vi "运维调试_氨氮.vi"() -> ()   [LabVIEW 2016, in "氨氮.lvlib"]
uses:
  <vilib>/Utility/miscctls.llb/LVPointTypeDef.ctl
  <vilib>/Utility/config.llb/NI_LVConfig.lvlib
panel:
  in  "质控参数设置":bool
  out "字符串":string
  in  "氨氮自动测试量程配置":T1
  out "ADC":sgl
  out "温度2":sgl
  out "温度1":sgl
  out "固件版本号":string
  in  "数组":string[](array[string])
  in  "备用系数写入":bool
  in  "备用系数读取":bool
  in  "备用系数":T2
  in  "量程切换阈值写入":bool
  in  "量程切换阈值读取":bool
  in  "量程切换阈值":cluster{"阈值":dbl, "标液浓度":dbl}
  in  "参数下拉列表":enum16{"氨氮", "总磷"}(ring)
  in  "量程下拉列表":enum16{"低量程", "高量程"}(ring)
  in  "测量模式下拉列表":enum16{"水样测量", "空白核查", "跨度核查", "标样核查", "加标回收"}(ring)
  in  "公式":cluster{"X^2":dbl, "X":dbl, "b":dbl}
  in  "写公式":bool
  in  "读公式":bool
  in  "精度":dbl=4.0
  in  "样品5 F0":dbl
  in  "样品5 F1":dbl
  in  "样品4 F1":dbl
  in  "样品4 F0":dbl
  in  "样品3 F0":dbl
  in  "样品3 F1":dbl
  in  "样品2 F0":dbl
  in  "样品2 F1":dbl
  in  "样品1 F1":dbl
  in  "样品1 F0":dbl
  in  "method":u16(ring) items=["最小二乘", "最小绝对残差", "Bisquare"]
  in  "模型":enum32{"线性", "多项式"}(ring)
  out "r^2":dbl format="%.7g"
  out "拟合公式":string
  in  "样品2启用":bool
  in  "样品5启用":bool
  in  "样品4启用":bool
  in  "样品3启用":bool
  in  "样品1启用":bool
  in  "标液浓度5":dbl
  in  "测量吸光度5":dbl
  in  "标液浓度4":dbl
  in  "测量吸光度4":dbl
  in  "标液浓度3":dbl
  in  "测量吸光度3":dbl
  in  "标液浓度2":dbl
  in  "测量吸光度2":dbl
  in  "测量吸光度1":dbl
  in  "标液浓度1":dbl
  out "XY图":cluster{"X Values":dbl[], "Y Values":dbl[]}[](graph)
  in  "返回":bool
  in  "设置":bool
  out "序列号":string="序列号"
  out "氨氮测量数据":T3(xcontrol)
  out "集成报警信息":string
  out "定时启动":bool
  out "总磷总氮运行状态":T4(xcontrol)
  in  "停止":bool
  in  "手动启动":bool
  in  "单步测试":bool
  in  "总磷氨氮调试":u16[](xcontrol)
  out "F3":sgl format="%#.6f"
  out "F2":sgl format="%#.6f"
  out "F1":sgl format="%#.6f"
  out "F0":sgl format="%#.6f"
  out "多列列表框":i32(listbox)
  # "参数设置"
  # "标液浓度"
  # "F0"
  # "F1"
  # "吸光值显示"
  # "样品一"
  # "辅\n助\n计\n算\n区"
  # "样品二"
  # "样品三"
  # "样品四"
  # "样品五"
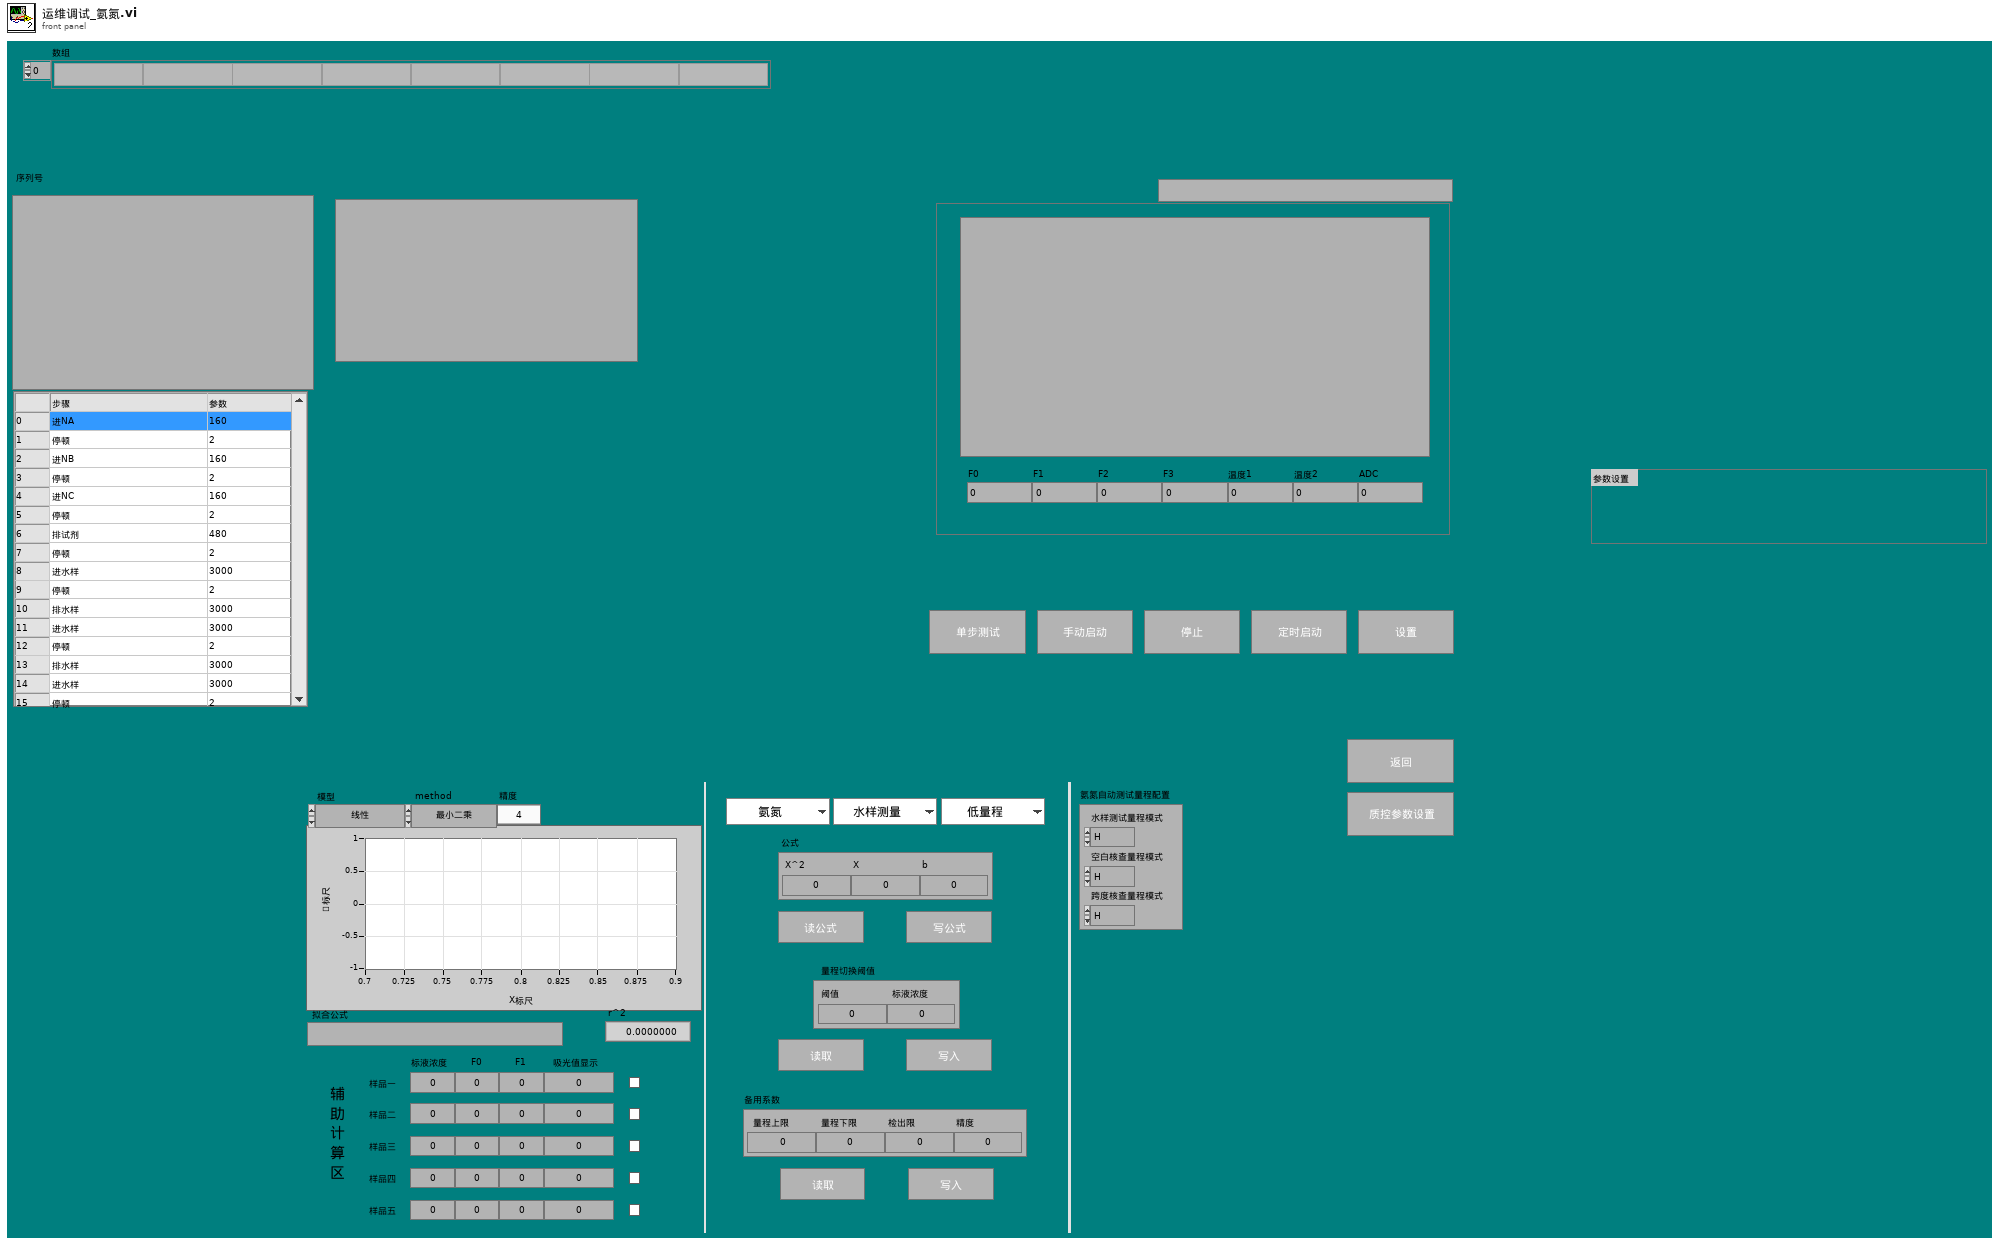
[diagram p1: front panel]
types:
  T1 = cluster{"水样测试量程模式":enum16{"H", "L", "AUTO"}, "空白核查量程模式":enum16{"H", "L", "AUTO"}, "跨度核查量程模式":enum16{"H", "L", "AUTO"}}
  T2 = cluster{"量程上限":dbl, "量程下限":dbl, "检出限":dbl, "精度":dbl}
  T3 = cluster{"flowid":u16, "测量精度":u16, "测量数据区":cluster{"因子编码":u32, "单位":u16, "标样参考值":sgl, "水样数据时间":timestamp, "水样实测值":sgl, "水样数据标识":string, "标样数据时间":timestamp, "标样实测值":sgl, "标样数据标识":string, "空白数据时间":timestamp, "空白实测值":sgl, "空白数据标识":string, "零点核查数据时间":timestamp, "零点核查实测值":sgl, "零点核查数据标识":string, "跨度核查数据时间":timestamp, "跨度核查实测值":sgl, "跨度核查数据标识":string, "加标回收数据时间":timestamp, "加标回收实测值":sgl, "加标回收数据标识":string, "平行样数据时间":timestamp, "平行样实测值":sgl, "平行样数据标识":string}}
  T4 = cluster{"系统时间":timestamp, "工作状态":enum16{"空闲", "水样测试", "标样核查", "零点核查", "跨度核查", "空白测试", "平行样测试", "加标回收", "空白校准", "标样校准", "初始化（清洗）"}, "测量模式":enum16{"待机", "连续模式", "周期模式", "定点模式", "受控模式", "手动模式"}, "告警代码":enum16{"无告警", "缺试剂告警", "缺水样告警", "缺蒸馏水告警", "缺标液告警", "仪表漏液告警", "标定异常告警", "超量程告警", "加热异常", "低试剂预警", "超上限告警", "超下限告警", "仪表内部其他异常", "滴定异常告警", "电极异常告警", "量程切换告警", "参数设置告警", "PH电极电位异常", "电导率电极异常", "浊度光度异常", "溶解氧电极异常", "溶解氧光强异常", "温度异常告警", "PH异常告警", "溶解氧异常告警", "电导率异常告警", "浊度异常告警", "叶绿素异常告警", "藻密度异常告警", "蓝绿藻异常告警", "ORP异常告警", "氨氮异常告警", "清洁刷异常告警", "SD卡异常告警", "蓝牙异常告警", "Wifi异常告警", "流程异常告警"}, "故障代码":enum16{"无故障", "电机故障", "温度故障", "通讯故障", "滴定故障"}, "日志代码":u16, "软件版本":u16, "F0":sgl, "F1":sgl, "F2":sgl, "F3":sgl, "T":sgl, "H":sgl, "id":u16, "flowid":u16, "量程":u16, "总磷控温温度1":sgl, "营养盐控温温度2":sgl, "ADC":sgl}
  T5 = cluster{"站号":u16, "量程切换":enum32{"H", "L", "AUTO"}, "控制命令":enum16{"启动测量", "标样核查", "零点核查", "跨度核查", "空白测试", "平行样测试", "加标回收", "空白校准", "标样校准", "初始化（清洗）", "停止测试", "仪器重启", "校时", "模式设置", "测量间隔设置"}, "模式设置":enum16{"待机", "连续模式", "周期模式", "定点模式", "受控模式", "手动模式"}, "测量间隔":u16}
  T6 = enum16{"启动测量", "标样核查", "零点核查", "跨度核查", "空白测试", "平行样测试", "加标回收", "空白校准", "标样校准", "初始化（清洗）", "停止测试", "仪器重启", "校时", "模式设置", "测量间隔设置"}
  T7 = cluster{"仪器测试类型":enum16{"水样测试", "标样核查", "空白测试", "跨度核查"}, "周期设置类型":enum16{"定点启动", "间隔启动"}, "定时功能启用":bool, "定时间隔":dbl, "24H周期设置":bool[]}
  T8 = enum32{"Bad", "Idle", "Run top level", "Running"}
  T9 = typedef "LVDateTimeRec.ctl" = cluster{"秒数的小数部分":dbl, "秒":i32, "分":i32, "时":i32, "日":i32, "月":i32, "年":i32, "天数（周）":i32, "天数（年）":i32, "DST":i32}
  T10 = typedef "LVPointTypeDef.ctl" = cluster{"Horizontal":i16, "Vertical":i16}
  T11 = cluster{"因子编码":u32, "单位":u16, "标样参考值":sgl, "水样数据时间":timestamp, "水样实测值":sgl, "水样数据标识":string, "标样数据时间":timestamp, "标样实测值":sgl, "标样数据标识":string, "空白数据时间":timestamp, "空白实测值":sgl, "空白数据标识":string, "零点核查数据时间":timestamp, "零点核查实测值":sgl, "零点核查数据标识":string, "跨度核查数据时间":timestamp, "跨度核查实测值":sgl, "跨度核查数据标识":string, "加标回收数据时间":timestamp, "加标回收实测值":sgl, "加标回收数据标识":string, "平行样数据时间":timestamp, "平行样实测值":sgl, "平行样数据标识":string}
  T12 = enum16{"空闲", "水样测试", "标样核查", "零点核查", "跨度核查", "空白测试", "平行样测试", "加标回收", "空白校准", "标样校准", "初始化（清洗）"}
  T13 = cluster{"启动模式":enum16{"标液测量", "水样测量", "零液测量", "盲样测量", "加标回收"}, "启动参数":u16, "量程":enum16{"低量程", "高量程"}}
  T14 = cluster{"时间标识":timestamp, "设备":string, "日志信息":string, "流程参数":string}
  T15 = cluster{"时间标识":timestamp, "设备":string, "日志信息":string}
  T16 = enum16{"无告警", "缺试剂告警", "缺水样告警", "缺蒸馏水告警", "缺标液告警", "仪表漏液告警", "标定异常告警", "超量程告警", "加热异常", "低试剂预警", "超上限告警", "超下限告警", "仪表内部其他异常", "滴定异常告警", "电极异常告警", "量程切换告警", "参数设置告警", "PH电极电位异常", "电导率电极异常", "浊度光度异常", "溶解氧电极异常", "溶解氧光强异常", "温度异常告警", "PH异常告警", "溶解氧异常告警", "电导率异常告警", "浊度异常告警", "叶绿素异常告警", "藻密度异常告警", "蓝绿藻异常告警", "ORP异常告警", "氨氮异常告警", "清洁刷异常告警", "SD卡异常告警", "蓝牙异常告警", "Wifi异常告警", "流程异常告警"}
  T17 = typedef "LVRowAndColumnUnsignedTypeDef.ctl" = cluster{"Row":u32, "Column":u32}
  T18 = typedef "NI_LVConfig.lvlib/Config Data RefNum.ctl" = refnum<k1>
  T19 = cluster{"XY图":cluster{"X Values":dbl[], "Y Values":dbl[]}[], "标液浓度1":dbl, "测量吸光度1":dbl, "测量吸光度2":dbl, "标液浓度2":dbl, "测量吸光度3":dbl, "标液浓度3":dbl, "测量吸光度4":dbl, "标液浓度4":dbl, "测量吸光度5":dbl, "标液浓度5":dbl, "样品1启用":bool, "样品3启用":bool, "样品4启用":bool, "样品5启用":bool, "样品2启用":bool, "拟合公式":string, "r^2":dbl, "模型":enum32{"线性", "多项式"}, "method":u16, "样品1 F0":dbl, "样品1 F1":dbl, "样品2 F1":dbl, "样品2 F0":dbl, "样品3 F1":dbl, "样品3 F0":dbl, "样品4 F0":dbl, "样品4 F1":dbl, "样品5 F1":dbl, "样品5 F0":dbl, "精度":dbl}
  T20 = cluster{"跨度值":dbl, "零点标准液浓度":dbl, "跨度标准液浓度":dbl, "标准液标准浓度":dbl}
  T21 = cluster{"确定":bool, "跨度值":dbl, "零点标准液浓度":dbl, "跨度标准液浓度":dbl, "标准液标准浓度":dbl}
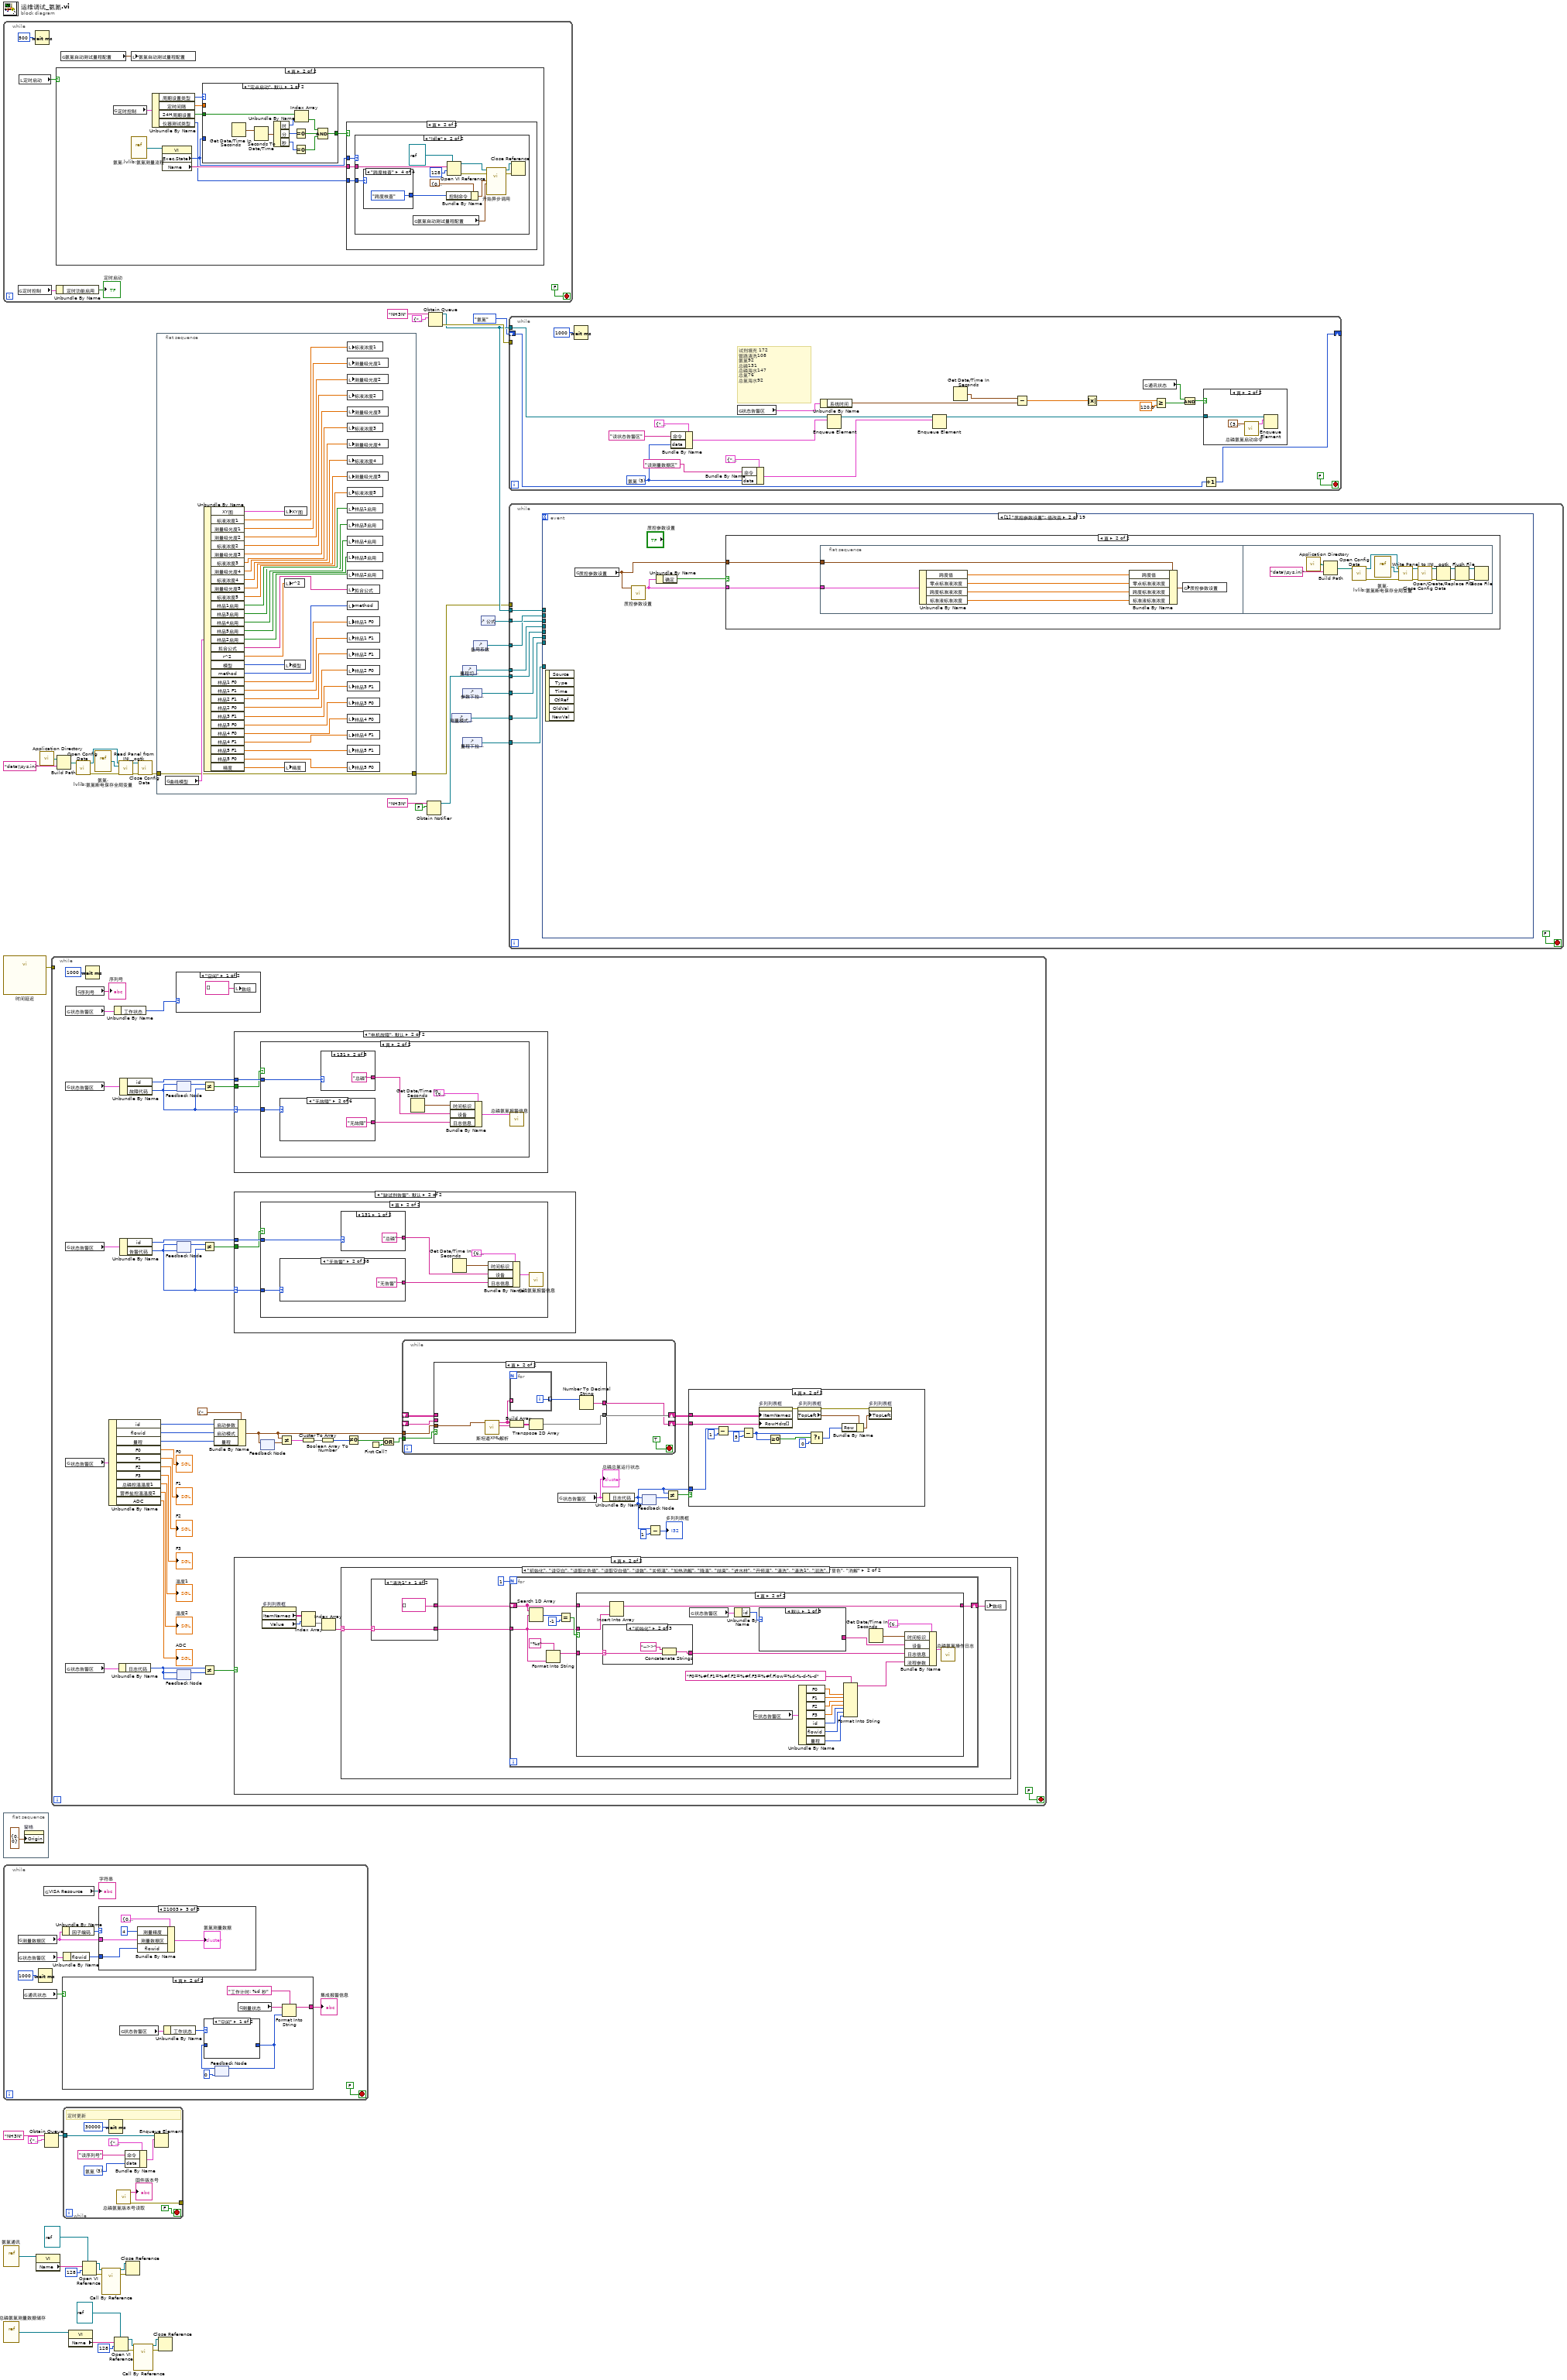
[diagram p0: block diagram]
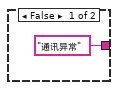
[diagram p2: hidden frame]
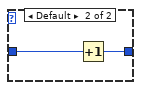
[diagram p3: hidden frame]
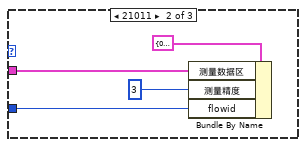
[diagram p5: hidden frame]
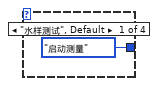
[diagram p9: hidden frame]
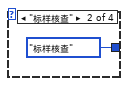
[diagram p10: hidden frame]
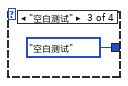
[diagram p11: hidden frame]
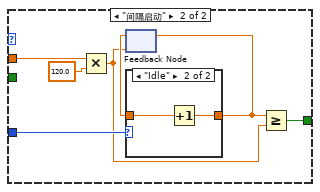
[diagram p12: hidden frame]
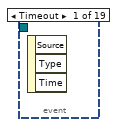
[diagram p14: hidden frame]
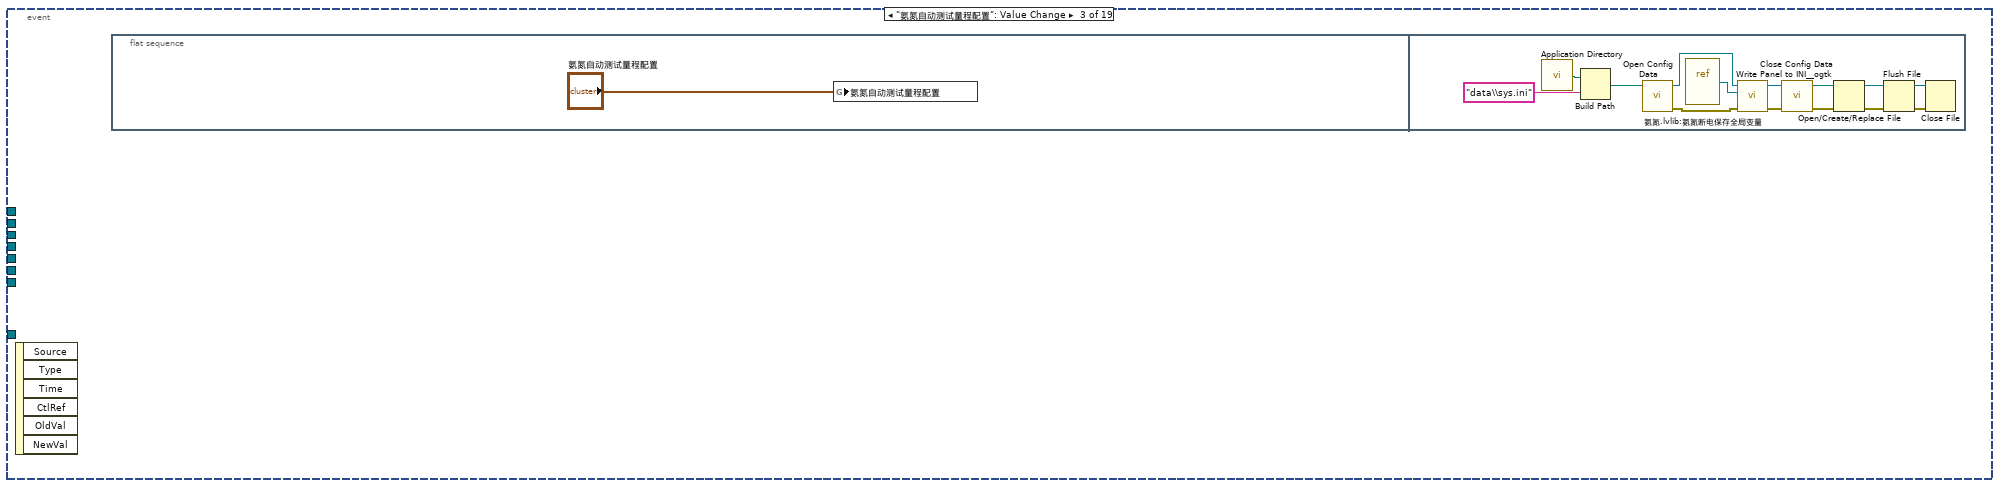
[diagram p16: hidden frame]
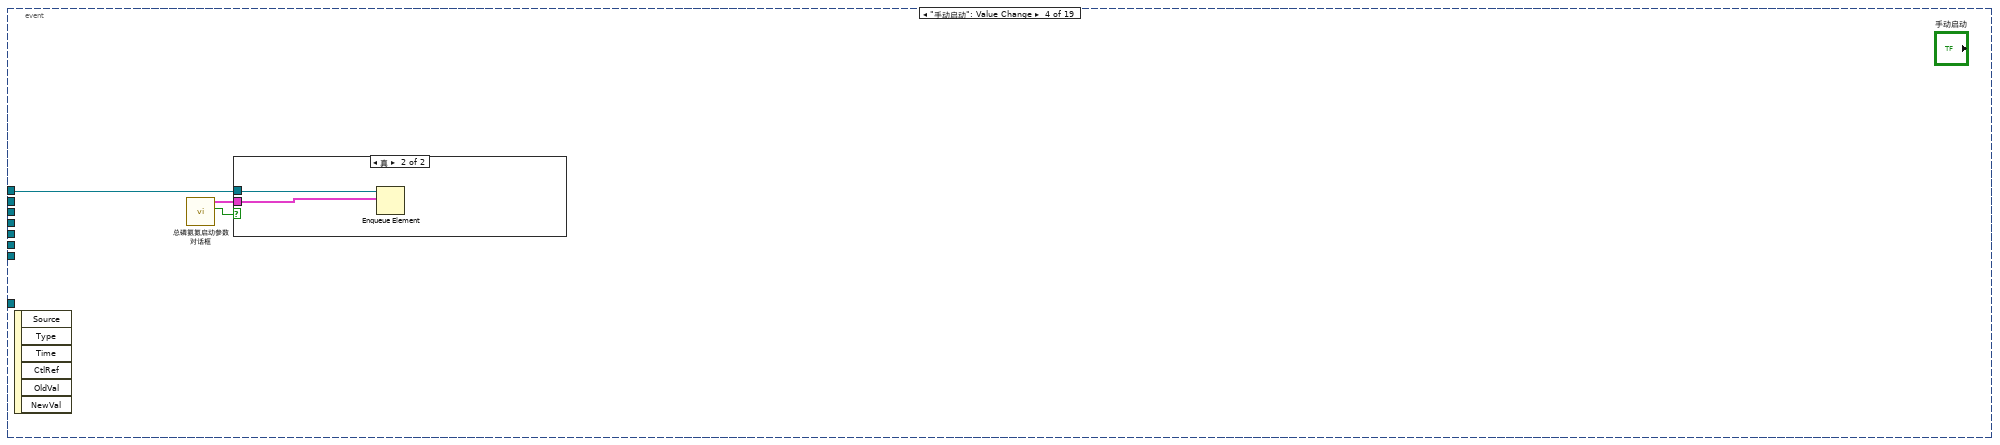
[diagram p17: hidden frame]
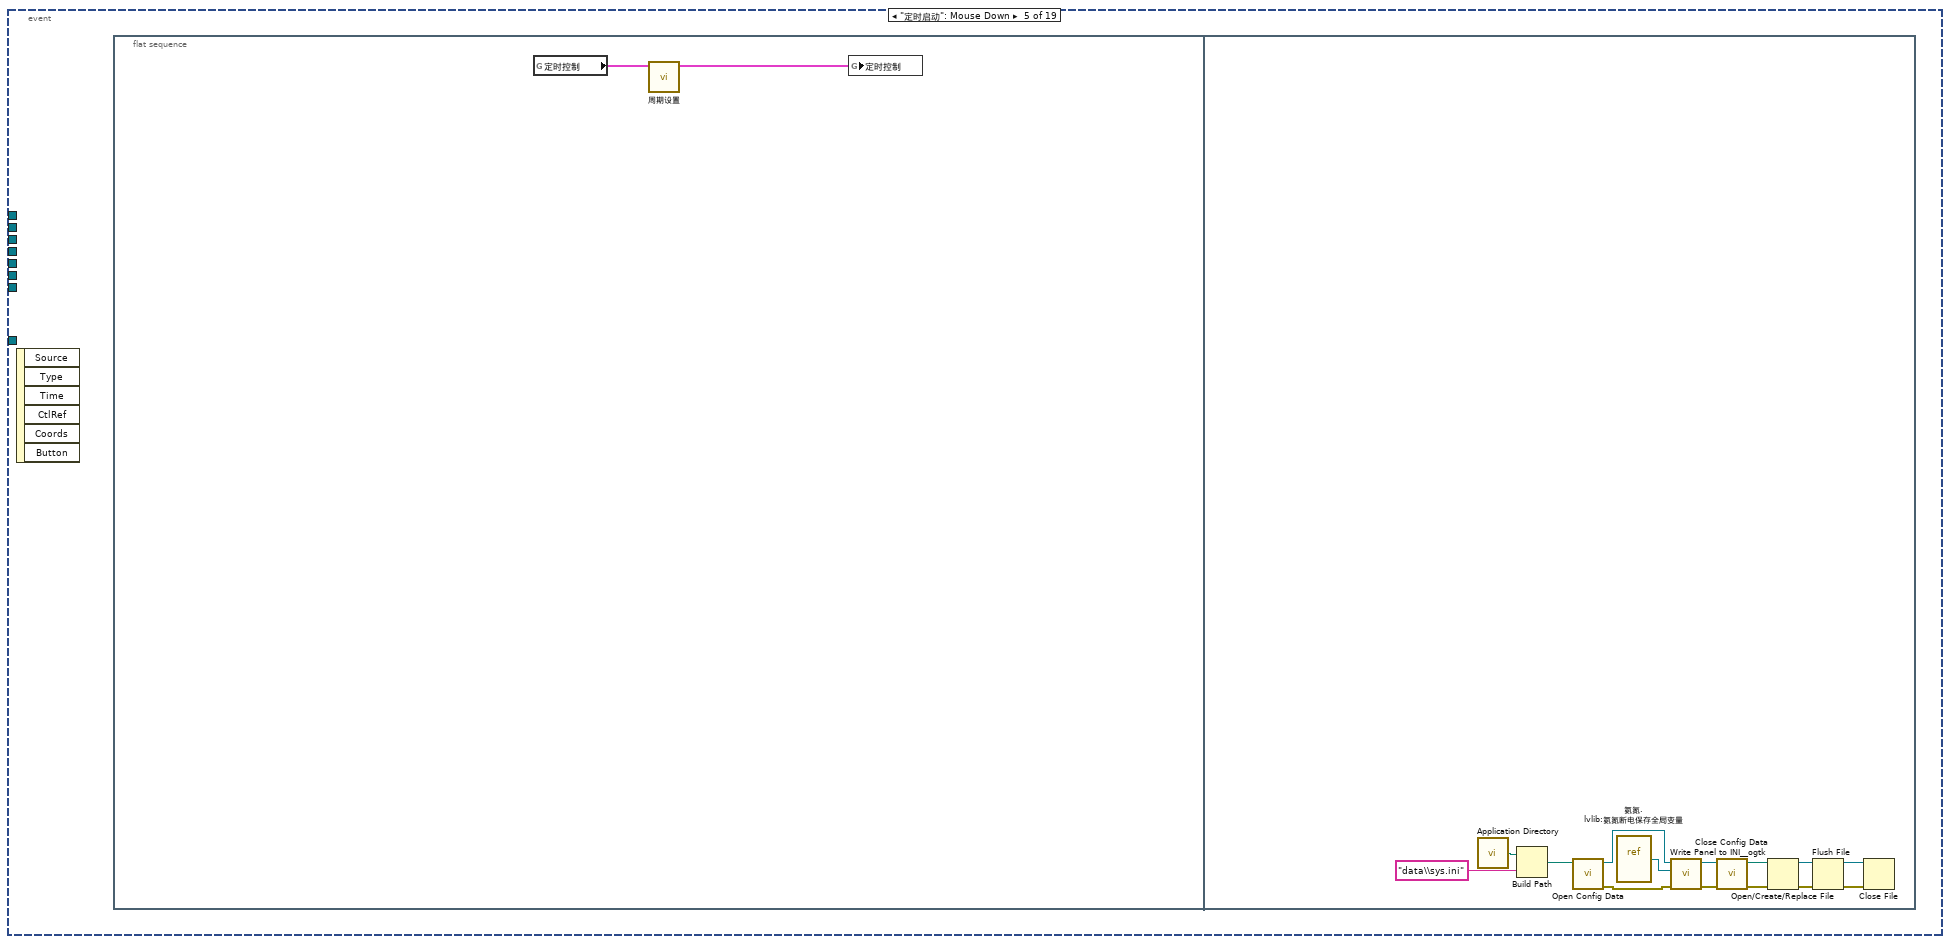
[diagram p19: hidden frame]
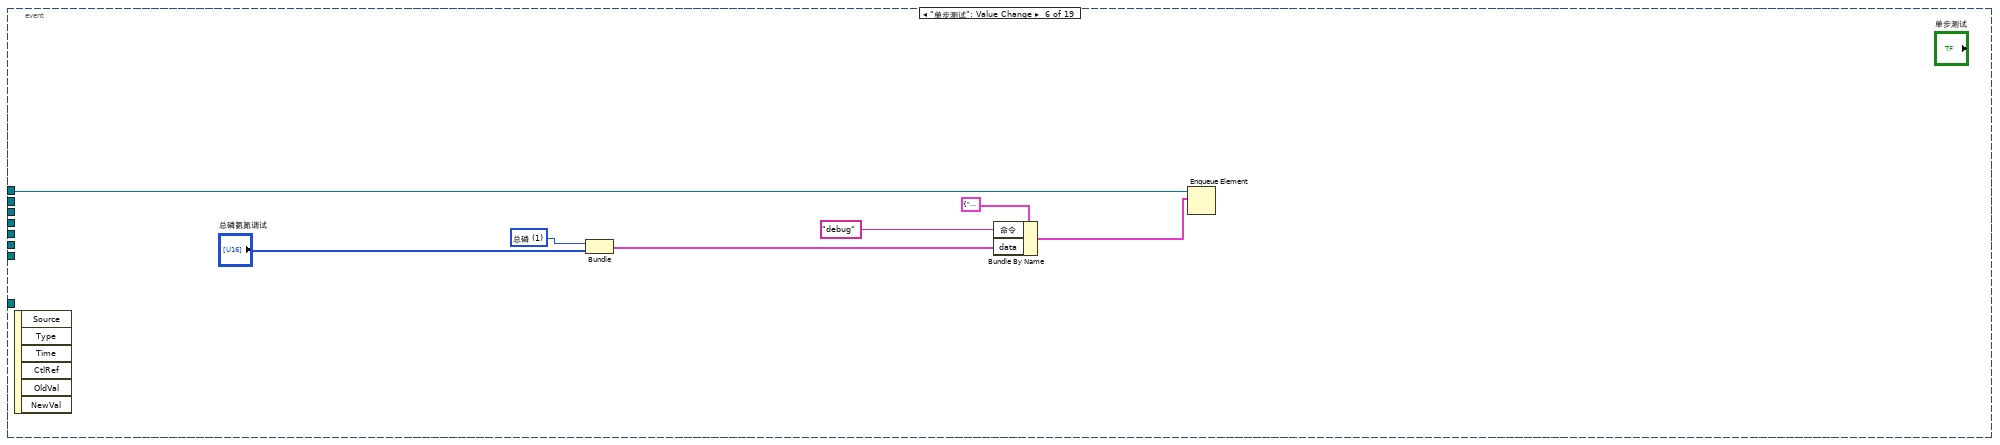
[diagram p20: hidden frame]
diagram:
  n1 = while {
    stop <- FALSE stop-if-true
    n2 = global read "氨氮断电保存全局变量.vi" "定时控制"() -> (w47:T7)
    n3 = local read "定时启动"() -> (w48:bool)
    n4 = Wait (ms)(milliseconds to wait=u32 500 ("等待时间（毫秒）")) -> ()  [unwired: 1 out]
    n5 = case shown="真" w48 {
      frame False {
      }
      frame True {
        n6 = global read "氨氮断电保存全局变量.vi" "定时控制"() -> (w59:T7)
        n7 = vi-ref "氨氮.lvlib:氨氮测量流程.vi"() -> (w55:refnum<vi>)
        n8 = Unbundle By Name(w59) -> ("周期设置类型"=w58:enum16{"定点启动", "间隔启动"}, "定时间隔"=w57:dbl, "24H周期设置"=w56:bool[], "仪器测试类型"=w52:enum16{"水样测试", "标样核查", "空白测试", "跨度核查"})
        n9 = property class="VI"(reference=w55) -> ("Exec.State"=w51:T8, "Name"=w54:string)  [unwired: 1 in, 2 out]
        n10 = case shown="\"定点启动\", 默认" w58 {
          tunnel: w57 -> [_ w92]
          tunnel: w56 -> [w88 _]
          tunnel: w51 -> [_ w95]
          tunnel: [w87 w90] -> w53
          frame "定点启动", Default {
            n11 = Get Date/Time In Seconds() -> (seconds since 1Jan1904=w86:timestamp)
            n12 = Seconds To Date/Time(time stamp (now)=w86) -> (date time rec=w85:T9)  [unwired: 1 in]
            n13 = Unbundle By Name(w85) -> ("时"=w84:i32, "分"=w82:i32, "秒"=w83:i32)
            n14 = Equal To 0?(x=w82) -> (x = 0?=w80:bool)
            n15 = Equal To 0?(x=w83) -> (x = 0?=w79:bool)
            n16 = Index Array(array=w88, index=w84) -> (element=w81:bool)
            n17 = Compound Arithmetic op=AND ("复合运算")(w81, w80, w79) -> (w87:bool)
          }
          frame "间隔启动" {
            n18 = Multiply(x=w92, y=120.0) -> (x*y=w89:dbl)
            n19 = feedback #1(w89) -> (w94:dbl)
            n20 = case shown="\"Idle\"" w95 {
              tunnel: w94 -> [_ w97]
              tunnel: [_ w96] -> w93
              frame "Bad", Default {
              }
              frame "Idle" {
                n21 = Increment(x=w97) -> (x+1=w96:dbl)
              }
            }
            n22 = feedback-in #1(w93) -> ()
            n23 = Greater Or Equal?(x=w93, y=w89) -> (x >= y?=w90:bool)
          }
        }
        n24 = case shown="真" w53 {
          tunnel: w54 -> [_ w62]
          tunnel: w52 -> [_ w61]
          tunnel: w51 -> [_ w60]
          frame False {
          }
          frame True {
            n25 = case shown="\"Idle\"" w60 {
              tunnel: w62 -> [_ w69]
              tunnel: w61 -> [_ w65]
              frame "Bad", Default {
              }
              frame "Idle" {
                n26 = case shown="\"跨度核查\"" w65 {
                  tunnel: [T6."启动测量" ("控制命令") T6."标样核查" ("控制命令") T6."空白测试" ("控制命令") T6."跨度核查" ("控制命令")] -> w64
                  frame "水样测试", Default {
                  }
                  frame "标样核查" {
                  }
                  frame "空白测试" {
                  }
                  frame "跨度核查" {
                  }
                }
                n27 = global read "氨氮断电保存全局变量.vi" "氨氮自动测试量程配置"() -> (w63:T1)
                n28 = Bundle By Name(cluster=T5 {"站号"=0, "量程切换"=enum."H", "控制命令"=enum."启动测量", "模式设置"=enum."待机", "测量间隔"=0} ("参数"), "控制命令"=w64) -> (w66:T5)
                n29 = Open VI Reference(type specifier VI Refnum (for type only)=refnum<vi> refnum, vi path=w69, options=128 ("选项")) -> (vi reference=w70:refnum<vi>, error out=w71:errorcluster)  [unwired: 3 in]
                n30 = call-by-ref "开始异步调用"(reference=w70, error in=w71, "量程模式"=w63, "参数"=w66) -> (reference out=w72:refnum<vi>, error out=w73:errorcluster)  [unwired: 10 in]
                n31 = Close Reference(reference=w72, error in (no error)=w73) -> ()  [unwired: 1 out]
              }
            }
          }
        }
      }
    }
    n32 = Unbundle By Name(w47) -> ("定时功能启用"=→"定时启动":bool)
    n33 = global read "氨氮断电保存全局变量.vi" "氨氮自动测试量程配置"() -> (w45:T1)
    n34 = local write "氨氮自动测试量程配置"(w45) -> ()
  }
  n35 = call "时间延迟"() -> ("error out"=w17:errorcluster)  [unwired: 11 in]
  n36 = flat-sequence {
    frame #0 {
      n37 = property on="窗格" class="Pane"("Origin"=T10 {"Horizontal"=0, "Vertical"=0} ("原点")) -> ()  [unwired: 2 in, 2 out]
    }
  }
  n38 = while {
    stop <- FALSE stop-if-true
    n39 = global read "VAR总磷氨氮全局变量.vi" "测量数据区"() -> (w105:T11)
    n40 = global read "VAR总磷氨氮全局变量.vi" "状态告警区"() -> (w101:T4)
    n41 = global read "VAR总磷氨氮全局变量.vi" "通讯状态"() -> (w103:bool)
    n42 = Wait (ms)(milliseconds to wait=u32 1000 ("等待时间（毫秒）")) -> ()  [unwired: 1 out]
    n43 = global read "VAR总磷氨氮全局变量.vi" "VISA Resource"() -> (→"字符串":refnum<visa-resource-name>)
    n44 = Unbundle By Name(w105) -> ("因子编码"=w104:u32)
    n45 = case shown="真" w103 {
      tunnel: ["通讯异常" ("集成报警信息") w110] -> w102
      frame False {
      }
      frame True {
        n46 = global read "VAR总磷氨氮全局变量.vi" "状态告警区"() -> (w116:T4)
        n47 = Unbundle By Name(w116) -> ("工作状态"=w115:T12)
        n48 = feedback #2(0) -> (w113:i32)
        n49 = case shown="\"空闲\"" w115 {
          tunnel: w113 -> [_ w118]
          tunnel: [_ w117] -> w111
          frame "空闲" {
          }
          frame Default {
            n50 = Increment(x=w118) -> (x+1=w117:i32)
          }
        }
        n51 = feedback-in #2(w111) -> ()
        n52 = global read "VAR总磷氨氮全局变量.vi" "测量状态"() -> (w109:string)
        n53 = Format Into String(format string="工作计时: %d 秒" ("格式字符串"), initial string=w109, w111) -> (resulting string=w110:string)  [unwired: 1 in, 1 out]
      }
    }
    "集成报警信息" <- w102
    n54 = Unbundle By Name(w101) -> ("flowid"=w100:u16)
    n55 = case shown="21003" w104 {
      tunnel: w105 -> [_ w122 w127]
      tunnel: w100 -> [_ w120 w125]
      frame Default {
      }
      frame 21011 {
        n56 = Bundle By Name(cluster=T3 {"flowid"=0, "测量精度"=0, "测量数据区"={"因子编码"=0, "单位"=0, "标样参考值"=0.0, "水样数据时间"=timestamp(0 s since 1904-01-01), "水样实测值"=0.0, "水样数据标识"="", "标样数据时间"=timestamp(0 s since 1904-01-01), "标样实测值"=0.0, "标样数据标识"="", "空白数据时间"=timestamp(0 s since 1904-01-01), "空白实测值"=0.0, "空白数据标识"="", "零点核查数据时间"=timestamp(0 s since 1904-01-01), "零点核查实测值"=0.0, "零点核查数据标识"="", "跨度核查数据时间"=timestamp(0 s since 1904-01-01), "跨度核查实测值"=0.0, "跨度核查数据标识"="", "加标回收数据时间"=timestamp(0 s since 1904-01-01), "加标回收实测值"=0.0, "加标回收数据标识"="", "平行样数据时间"=timestamp(0 s since 1904-01-01), "平行样实测值"=0.0, "平行样数据标识"=""}} ("氨氮测量数据"), "测量数据区"=w122, "测量精度"=u16 3, "flowid"=w120) -> ()  [unwired: 1 out]
      }
      frame 21003 {
        n57 = Bundle By Name(cluster=T3 {"flowid"=0, "测量精度"=0, "测量数据区"={"因子编码"=0, "单位"=0, "标样参考值"=0.0, "水样数据时间"=timestamp(0 s since 1904-01-01), "水样实测值"=0.0, "水样数据标识"="", "标样数据时间"=timestamp(0 s since 1904-01-01), "标样实测值"=0.0, "标样数据标识"="", "空白数据时间"=timestamp(0 s since 1904-01-01), "空白实测值"=0.0, "空白数据标识"="", "零点核查数据时间"=timestamp(0 s since 1904-01-01), "零点核查实测值"=0.0, "零点核查数据标识"="", "跨度核查数据时间"=timestamp(0 s since 1904-01-01), "跨度核查实测值"=0.0, "跨度核查数据标识"="", "加标回收数据时间"=timestamp(0 s since 1904-01-01), "加标回收实测值"=0.0, "加标回收数据标识"="", "平行样数据时间"=timestamp(0 s since 1904-01-01), "平行样实测值"=0.0, "平行样数据标识"=""}} ("氨氮测量数据"), "测量精度"=u16 4, "测量数据区"=w127, "flowid"=w125) -> (→"氨氮测量数据":T3)
      }
    }
  }
  n58 = vi-ref "氨氮通讯.vi"() -> (w40:refnum<vi>)
  n59 = vi-ref "总磷氨氮测量数据储存.vi"() -> (w32:refnum<vi>)
  n60 = property class="VI"(reference=w40) -> ("Name"=w39:string)  [unwired: 1 in, 2 out]
  n61 = call <vilib>:"Application Directory.vi"() -> ("Application Directory"=w3:path)
  n62 = Obtain Queue(name (unnamed)="NH3N" ("名称（未命名）"), element data type=cluster{"命令":string, "data":variant} {"命令"="", "data"=variant}) -> (queue out=w14:refnum<queue>)  [unwired: 3 in, 2 out]
  n63 = while {
    tunnel: w17 -> [_]
    stop <- FALSE stop-if-true
    n64 = global read "VAR总磷氨氮全局变量.vi" "状态告警区"() -> (w139:T4)
    n65 = global read "VAR总磷氨氮全局变量.vi" "状态告警区"() -> (w144:T4)
    n66 = global read "VAR总磷氨氮全局变量.vi" "状态告警区"() -> (w149:T4)
    n67 = global read "VAR总磷氨氮全局变量.vi" "状态告警区"() -> (w161:T4)
    n68 = global read "VAR总磷氨氮全局变量.vi" "状态告警区"() -> (w136:T4)
    n69 = global read "VAR总磷氨氮全局变量.vi" "序列号"() -> (→"序列号":string)
    n70 = Wait (ms)(milliseconds to wait=u32 1000 ("等待时间（毫秒）")) -> ()  [unwired: 1 out]
    n71 = Unbundle By Name(w161) -> ("id"=w158:u16, "flowid"=w160:u16, "量程"=w159:u16, "F0"=→"F0":sgl, "F1"=→"F1":sgl, "F2"=→"F2":sgl, "F3"=→"F3":sgl, "总磷控温温度1"=→"温度1":sgl, "营养盐控温温度2"=→"温度2":sgl, "ADC"=→"ADC":sgl)
    n72 = Unbundle By Name(w139) -> ("工作状态"=w138:T12)
    n73 = Unbundle By Name(w136) -> ("日志代码"=w135:u16)
    n74 = Unbundle By Name(w144) -> ("id"=w143:u16, "故障代码"=w140:enum16{"无故障", "电机故障", "温度故障", "通讯故障", "滴定故障"})
    n75 = Unbundle By Name(w149) -> ("id"=w148:u16, "告警代码"=w145:T16)
    n76 = case shown="\"空闲\"" w138 {
      frame "空闲" {
        n77 = local write "数组"(string[] [] ("数组")) -> ()
      }
      frame "水样测试", Default {
      }
    }
    n78 = feedback #3(w140) -> (w141:enum16{"无故障", "电机故障", "温度故障", "通讯故障", "滴定故障"})
    n79 = feedback-in #3(w140) -> ()
    n80 = feedback #4(w145) -> (w146:T16)
    n81 = feedback-in #4(w145) -> ()
    n82 = feedback #5(w135) -> (w137:u16)
    n83 = feedback-in #5(w135) -> ()
    n84 = Not Equal?(x=w141, y=w140) -> (x != y?=w142:bool)
    n85 = Not Equal?(x=w146, y=w145) -> (x != y?=w147:bool)
    n86 = Not Equal?(x=w135, y=w137) -> (x != y?=w134:bool)
    n87 = Bundle By Name(cluster=T13 {"启动模式"=enum."加标回收", "启动参数"=1, "量程"=enum."低量程"} ("参数簇"), "启动参数"=w158, "启动模式"=w160, "量程"=w159) -> (w151:T13)
    n88 = case shown="\"电机故障\", 默认" w140 {
      selector: w140 -> [_ w229]
      tunnel: w143 -> [_ w230]
      tunnel: w142 -> [_ w228]
      frame "无故障" {
      }
      frame "电机故障", Default {
        n89 = case shown="真" w228 {
          tunnel: w230 -> [_ w237]
          tunnel: w229 -> [_ w232]
          frame False {
          }
          frame True {
            n90 = case shown="\"无故障\"" w232 {
              selector: w232 -> [w239 _ _ _ _ _]
              tunnel: [w238 "无故障" "电机故障" "温度故障" "通讯故障" "滴定故障"] -> w231
              frame Default {
                n91 = Format Into String(format string="%d" ("格式字符串"), initial string="未知" ("工作状态"), w239) -> (resulting string=w238:string)  [unwired: 1 in, 1 out]
              }
              frame "无故障" {
              }
              frame "电机故障" {
              }
              frame "温度故障" {
              }
              frame "通讯故障" {
              }
              frame "滴定故障" {
              }
            }
            n92 = case shown="131" w237 {
              tunnel: [_ "总磷" ("table输入") "氨氮" ("table输入")] -> w233
              frame Default {
              }
              frame 131 {
              }
              frame 92 {
              }
            }
            n93 = Get Date/Time In Seconds() -> (seconds since 1Jan1904=w234:timestamp)
            n94 = Bundle By Name(cluster=T15 {"时间标识"=timestamp(0 s since 1904-01-01), "设备"="", "日志信息"=""} ("data in"), "时间标识"=w234, "设备"=w233, "日志信息"=w231) -> (w235:T15)
            n95 = call "总磷氨氮报警信息.vi"("data in"=w235) -> ()  [unwired: 11 in]
          }
        }
      }
    }
    n96 = case shown="\"缺试剂告警\", 默认" w145 {
      selector: w145 -> [_ w250]
      tunnel: w148 -> [_ w251]
      tunnel: w147 -> [_ w249]
      frame "无告警" {
      }
      frame "缺试剂告警", Default {
        n97 = case shown="真" w249 {
          tunnel: w251 -> [_ w258]
          tunnel: w250 -> [_ w252]
          frame False {
          }
          frame True {
            n98 = case shown="\"无告警\"" w252 {
              selector: w252 -> [w260 _ _ _ _ _ _ _ _ _ _ _ _ _ _ _ _ _ _ _ _ _ _ _ _ _ _ _ _ _ _ _ _ _ _ _ _ _]
              tunnel: [w259 "无告警" "缺试剂告警" "缺水样告警" "缺蒸馏水告警" "缺标液告警" "仪表漏液告警" "标定异常告警" "超量程告警" "加热异常" "低试剂预警" "超上限告警" "超下限告警" "仪表内部其他异常" "滴定异常告警" "电极异常告警" "量程切换告警" "参数设置告警" "PH电极电位异常" "电导率电极异常" "浊度光度异常" "溶解氧电极异常" "溶解氧光强异常" "温度异常告警" "PH异常告警" "溶解氧异常告警" "电导率异常告警" "浊度异常告警" "叶绿素异常告警" "藻密度异常告警" "蓝绿藻异常告警" "ORP异常告警" "氨氮异常告警" "清洁刷异常告警" "SD卡异常告警" "蓝牙异常告警" "WiFi异常告警" "流程异常告警"] -> w253
              frame Default {
                n99 = Format Into String(format string="%d" ("格式字符串"), initial string="未知" ("工作状态"), w260) -> (resulting string=w259:string)  [unwired: 1 in, 1 out]
              }
              frame "无告警" {
              }
              frame "缺试剂告警" {
              }
              frame "缺水样告警" {
              }
              frame "缺蒸馏水告警" {
              }
              frame "缺标液告警" {
              }
              frame "仪表漏液告警" {
              }
              frame "标定异常告警" {
              }
              frame "超量程告警" {
              }
              frame "加热异常" {
              }
              frame "低试剂预警" {
              }
              frame "超上限告警" {
              }
              frame "超下限告警" {
              }
              frame "仪表内部其他异常" {
              }
              frame "滴定异常告警" {
              }
              frame "电极异常告警" {
              }
              frame "量程切换告警" {
              }
              frame "参数设置告警" {
              }
              frame "PH电极电位异常" {
              }
              frame "电导率电极异常" {
              }
              frame "浊度光度异常" {
              }
              frame "溶解氧电极异常" {
              }
              frame "溶解氧光强异常" {
              }
              frame "温度异常告警" {
              }
              frame "PH异常告警" {
              }
              frame "溶解氧异常告警" {
              }
              frame "电导率异常告警" {
              }
              frame "浊度异常告警" {
              }
              frame "叶绿素异常告警" {
              }
              frame "藻密度异常告警" {
              }
              frame "蓝绿藻异常告警" {
              }
              frame "ORP异常告警" {
              }
              frame "氨氮异常告警" {
              }
              frame "清洁刷异常告警" {
              }
              frame "SD卡异常告警" {
              }
              frame "蓝牙异常告警" {
              }
              frame "Wifi异常告警" {
              }
              frame "流程异常告警" {
              }
            }
            n100 = case shown="131" w258 {
              tunnel: ["总磷" ("table输入") "氨氮" ("table输入")] -> w254
              frame 131 {
              }
              frame 92, Default {
              }
            }
            n101 = Get Date/Time In Seconds() -> (seconds since 1Jan1904=w255:timestamp)
            n102 = Bundle By Name(cluster=T15 {"时间标识"=timestamp(0 s since 1904-01-01), "设备"="", "日志信息"=""} ("data in"), "时间标识"=w255, "设备"=w254, "日志信息"=w253) -> (w256:T15)
            n103 = call "总磷氨氮报警信息.vi"("data in"=w256) -> ()  [unwired: 11 in]
          }
        }
      }
    }
    n104 = case shown="真" w134 {
      frame False {
      }
      frame True {
        n105 = property on="多列列表框" class="MCListbox (严格)"() -> ("ItemNames"=w178:string[][], "Value"=w179:i32)  [unwired: 2 in, 2 out]
        n106 = Index Array(array=w178, index (row)=w179) -> (element=w177:string[])  [unwired: 1 in]
        n107 = Index Array(array=w177) -> (element=w176:string)  [unwired: 1 in]
        n108 = case shown="\"初始化\", \"读空白\", \"读取比色值\", \"读取空白值\", \"读数\", \"关恒温\", \"加热消解\", \"降温\", \"结束\", \"进水样\", \"开恒温\", \"清洗\", \"清洗1\", \"润洗\", \"显色\", \"消解\"" w176 {
          selector: w176 -> [_ w182]
          frame Default {
          }
          frame "初始化", "读空白", "读取比色值", "读取空白值", "读数", "关恒温", "加热消解", "降温", "结束", "进水样", "开恒温", "清洗", "清洗1", "润洗", "显色", "消解" {
            n109 = case shown="\"清洗1\"" w182 {
              selector: w182 -> [w186 w188]
              tunnel: [w186 w188] -> w181
              tunnel: [string[] [] ("数组") "数组"] -> w180
              frame "清洗1" {
              }
              frame Default {
              }
            }
            n110 = for {
              N: 1 -> [_]
              tunnel: w181 -> [w190]
              shift-right: [w189] -> w183
              shift-left: w180 -> [w191]
              n111 = Search 1D Array(1D array=w191, element=w190) -> (index of element=w194:i32)  [unwired: 1 in]
              n112 = Format Into String(format string="%s" ("格式字符串"), w190) -> (resulting string=w195:string)  [unwired: 2 in, 1 out]
              n113 = Equal?(x=w194, y=-1) -> (x = y?=w192:bool)
              n114 = case shown="真" w192 {
                tunnel: w195 -> [_ w199]
                tunnel: w191 -> [w197 w203]
                tunnel: w190 -> [_ w202]
                tunnel: [w197 w201] -> w189
                frame False {
                }
                frame True {
                  n115 = case shown="\"初始化\"" w199 {
                    selector: w199 -> [w219 w222 w225]
                    tunnel: [w219 w221 w224] -> w198
                    frame Default {
                    }
                    frame "初始化" {
                      n116 = Concatenate Strings("-->>" ("字符串"), w222) -> (w221:string)
                    }
                    frame "结束" {
                      n117 = Concatenate Strings("-->>" ("字符串"), w225) -> (w224:string)
                    }
                  }
                  n118 = Insert Into Array(array=w203, new element=w202) -> (w201:string[])  [unwired: 1 in]
                  n119 = global read "VAR总磷氨氮全局变量.vi" "状态告警区"() -> (w218:T4)
                  n120 = Unbundle By Name(w218) -> ("id"=w217:u16)
                  n121 = global read "VAR总磷氨氮全局变量.vi" "状态告警区"() -> (w213:T4)
                  n122 = case shown="默认" w217 {
                    tunnel: [_ "总磷" ("table输入") "氨氮" ("table输入")] -> w215
                    frame Default {
                    }
                    frame 131 {
                    }
                    frame 92 {
                    }
                  }
                  n123 = Unbundle By Name(w213) -> ("F0"=w210:sgl, "F1"=w209:sgl, "F2"=w208:sgl, "F3"=w207:sgl, "id"=w206:u16, "flowid"=w205:u16, "量程"=w204:u16)
                  n124 = Format Into String(format string="F0=%#f,F1=%#f,F2=%#f,F3=%#f,Flow=%d-%-d-%-d" ("格式字符串"), w210, w209, w208, w207, w206, w205, w204) -> (resulting string=w211:string)  [unwired: 2 in, 1 out]
                  n125 = Get Date/Time In Seconds() -> (seconds since 1Jan1904=w214:timestamp)
                  n126 = Bundle By Name(cluster=T14 {"时间标识"=timestamp(0 s since 1904-01-01), "设备"="", "日志信息"="", "流程参数"=""} ("data in"), "时间标识"=w214, "设备"=w215, "日志信息"=w198, "流程参数"=w211) -> (w216:T14)
                  n127 = call "总磷氨氮操作日志.vi"("data in"=w216) -> ()  [unwired: 11 in]
                }
              }
            }
            n128 = local write "数组"(w183) -> ()
          }
        }
      }
    }
    n129 = feedback #6() -> (w167:T13)  [unwired: 1 in]
    n130 = feedback-in #6(w151) -> ()
    n131 = Not Equal?(x=w151, y=w167) -> (x != y?=w168:cluster{"启动模式":bool, "启动参数":bool, "量程":bool})
    n132 = Cluster To Array(cluster=w168) -> (array=w169:bool[])
    n133 = Boolean Array To Number(Boolean array=w169) -> (number=w170:u32)
    n134 = Not Equal To 0?(x=w170) -> (x != 0?=w163:bool)
    n135 = First Call?() -> (First Call?: T/F=w164:bool)
    n136 = Or(x=w163, y=w164) -> (x .or. y?=w162:bool)
    n137 = while {
      tunnel: w162 -> [w308]
      tunnel: w151 -> [w307]
      shift-right: [w306] -> w166
      shift-left: _ -> [w302]
      shift-right: [w305] -> w165
      shift-left: _ -> [w303]
      stop <- TRUE stop-if-true
      n138 = case shown="真" w308 {
        tunnel: [w310 w317] -> w305
        tunnel: [w309 w316] -> w306
        tunnel: w307 -> [_ w311]
        tunnel: w303 -> [w310 _]
        tunnel: w302 -> [w309 _]
        frame False {
        }
        frame True {
          n139 = call "斯坦道XML解析.vi"("参数簇"=w311) -> ("步骤时间"=w312:string[], "步骤名"=w314:string[])  [unwired: 9 in]
          n140 = for {
            tunnel: w314 -> [_] mode=indexing
            tunnel: [w318] -> w315 mode=indexing
            i -> [w318]
          }
          n141 = Build Array(w314, w312) -> (w313:string[][])
          n142 = Transpose 2D Array(2D array=w313) -> (transposed array=w316:string[][])
          n143 = Number To Decimal String(number=w315) -> (decimal integer string=w317:string[])  [unwired: 1 in]
        }
      }
    }
    n144 = global read "VAR总磷氨氮全局变量.vi" "状态告警区"() -> (w152:T4)
    "总磷总氮运行状态" <- w152
    n145 = Unbundle By Name(w152) -> ("日志代码"=w129:u16)
    n146 = feedback-in #7(w129) -> ()
    n147 = feedback #7(w129) -> (w172:u16)
    n148 = Subtract(x=w129, y=1) -> (x-y=→"多列列表框":i32)
    n149 = Not Equal?(x=w129, y=w172) -> (x != y?=w171:bool)
    n150 = case shown="真" w171 {
      tunnel: w129 -> [_ w321]
      tunnel: w166 -> [_ w328]
      tunnel: w165 -> [_ w327]
      frame False {
      }
      frame True {
        n151 = Subtract(x=w321, y=1) -> (x-y=w319:i32)
        n152 = Subtract(x=w319, y=5) -> (x-y=w323:i32)
        n153 = property on="多列列表框" class="MCListbox (严格)"("ItemNames"=w328, "RowHdrs[]"=w327) -> (error out=w329:errorcluster)  [unwired: 2 in, 1 out]
        n154 = Greater Or Equal To 0?(x=w323) -> (x >= 0?=w322:bool)
        n155 = property on="多列列表框" class="MCListbox (严格)"(error in=w329) -> (error out=w330:errorcluster, "TopLeft"=w331:T17)  [unwired: 1 in, 1 out]
        n156 = Select(t=w323, s=w322, f=0) -> (s? t:f=w324:i32)
        n157 = Bundle By Name(cluster=w331, "Row"=w324) -> (w332:T17)
        n158 = property on="多列列表框" class="MCListbox (严格)"(error in=w330, "TopLeft"=w332) -> ()  [unwired: 1 in, 2 out]
      }
    }
  }
  n159 = Build Path(base path=w3, name or relative path="data\\sys.ini" ("名称或相对路径")) -> (appended path=w5:path)
  n160 = while {
    tunnel: w14 -> [w337]
    tunnel: [w334] -> _
    stop <- FALSE stop-if-true
    w338 = u16 3 items=["总磷"=1, "氨氮"=3] ("站号")
    # "定时更新"
    n161 = Wait (ms)(milliseconds to wait=u32 30000 ("等待时间（毫秒）")) -> ()  [unwired: 1 out]
    n162 = call "总磷氨氮版本号读取.vi"() -> ("error out"=w334:errorcluster, "固件版本号"=→"固件版本号":string)  [unwired: 10 in]
    n163 = Bundle By Name(cluster=cluster{"命令":string, "data":variant} {"命令"="", "data"=variant} ("元素"), "命令"="读序列号", "data"=w338) -> (w336:cluster{"命令":string, "data":variant})
    n164 = Enqueue Element(queue=w337, element=w336) -> ()  [unwired: 2 in, 3 out]
  }
  n165 = property class="VI"(reference=w32) -> ("Name"=w25:string)  [unwired: 1 in, 2 out]
  n166 = call <vilib>:"Open Config Data.vi"("configuration file path"=w5) -> ("error out"=w9:errorcluster, "refnum"=w6:T18)  [unwired: 8 in, 1 out]
  n167 = Open VI Reference(type specifier VI Refnum (for type only)=refnum<vi> refnum, vi path=w39, options=128 ("选项")) -> (vi reference=w37:refnum<vi>, error out=w35:errorcluster)  [unwired: 3 in]
  n168 = vi-ref "氨氮.lvlib:氨氮断电保存全局变量.vi"() -> (w7:refnum<vi>)
  n169 = call-by-ref "?"(reference=w37, error in=w35) -> (reference out=w33:refnum<vi>, error out=w34:errorcluster)  [unwired: 12 in]
  n170 = Open VI Reference(type specifier VI Refnum (for type only)=refnum<vi> refnum, vi path=w25, options=128 ("选项")) -> (vi reference=w27:refnum<vi>, error out=w29:errorcluster)  [unwired: 3 in]
  n171 = call <userlib>:"Read Panel from INI__ogtk.vi"("error in (no error)"=w9, "VI ref"=w7, "refnum"=w6) -> ("error out"=w10:errorcluster, "refnum out"=w8:T18)  [unwired: 7 in]
  n172 = Close Reference(reference=w33, error in (no error)=w34) -> ()  [unwired: 1 out]
  n173 = call-by-ref "?"(reference=w27, error in=w29) -> (reference out=w31:refnum<vi>, error out=w30:errorcluster)  [unwired: 12 in]
  n174 = call <vilib>:"Close Config Data.vi"("error in (no error)"=w10, "refnum"=w8) -> ("error out"=w2:errorcluster)  [unwired: 8 in, 1 out]
  n175 = flat-sequence {
    tunnel: w2 -> [w342]
    tunnel: [w342] -> w1
    frame #0 {
      n176 = global read "氨氮断电保存全局变量.vi" "曲线模型"() -> (w374:T19)
      n177 = Unbundle By Name(w374) -> ("XY图"=w373:cluster{"X Values":dbl[], "Y Values":dbl[]}[], "标液浓度1"=w372:dbl, "测量吸光度1"=w371:dbl, "测量吸光度2"=w370:dbl, "标液浓度2"=w369:dbl, "测量吸光度3"=w368:dbl, "标液浓度3"=w367:dbl, "测量吸光度4"=w366:dbl, "标液浓度4"=w365:dbl, "测量吸光度5"=w364:dbl, "标液浓度5"=w363:dbl, "样品1启用"=w362:bool, "样品3启用"=w360:bool, "样品4启用"=w359:bool, "样品5启用"=w358:bool, "样品2启用"=w361:bool, "拟合公式"=w357:string, "r^2"=w356:dbl, "模型"=w355:enum32{"线性", "多项式"}, "method"=w354:u16, "样品1 F0"=w353:dbl, "样品1 F1"=w352:dbl, "样品2 F1"=w351:dbl, "样品2 F0"=w350:dbl, "样品3 F1"=w349:dbl, "样品3 F0"=w348:dbl, "样品4 F0"=w347:dbl, "样品4 F1"=w346:dbl, "样品5 F1"=w345:dbl, "样品5 F0"=w344:dbl, "精度"=w343:dbl)
      n178 = local write "XY图"(w373) -> ()
      n179 = local write "r^2"(w356) -> ()
      n180 = local write "模型"(w355) -> ()
      n181 = local write "精度"(w343) -> ()
      n182 = local write "标液浓度1"(w372) -> ()
      n183 = local write "测量吸光度1"(w371) -> ()
      n184 = local write "测量吸光度2"(w370) -> ()
      n185 = local write "标液浓度2"(w369) -> ()
      n186 = local write "测量吸光度3"(w368) -> ()
      n187 = local write "标液浓度3"(w367) -> ()
      n188 = local write "测量吸光度4"(w366) -> ()
      n189 = local write "标液浓度4"(w365) -> ()
      n190 = local write "测量吸光度5"(w364) -> ()
      n191 = local write "标液浓度5"(w363) -> ()
      n192 = local write "样品1启用"(w362) -> ()
      n193 = local write "样品3启用"(w360) -> ()
      n194 = local write "样品4启用"(w359) -> ()
      n195 = local write "样品5启用"(w358) -> ()
      n196 = local write "样品2启用"(w361) -> ()
      n197 = local write "拟合公式"(w357) -> ()
      n198 = local write "method"(w354) -> ()
      n199 = local write "样品1 F0"(w353) -> ()
      n200 = local write "样品1 F1"(w352) -> ()
      n201 = local write "样品2 F1"(w351) -> ()
      n202 = local write "样品2 F0"(w350) -> ()
      n203 = local write "样品3 F1"(w349) -> ()
      n204 = local write "样品3 F0"(w348) -> ()
      n205 = local write "样品4 F0"(w347) -> ()
      n206 = local write "样品4 F1"(w346) -> ()
      n207 = local write "样品5 F1"(w345) -> ()
      n208 = local write "样品5 F0"(w344) -> ()
    }
  }
  n209 = Close Reference(reference=w31, error in (no error)=w30) -> ()  [unwired: 1 out]
  n210 = Obtain Notifier(name (unnamed)="NH3N" ("名称（未命名）"), notification data type=FALSE) -> (notifier out=w11:refnum<notifier>)  [unwired: 2 in, 2 out]
  n211 = Obtain Queue(name (unnamed)="NH3N" ("名称（未命名）"), element data type=cluster{"命令":string, "data":variant} {"命令"="", "data"=variant}) -> (queue out=w41:refnum<queue>, error out=w42:errorcluster)  [unwired: 3 in, 1 out]
  n212 = control-ref of="测量模式下拉列表"() -> (w21:refnum<vi>)
  n213 = control-ref of="量程切换阈值"() -> (w19:refnum<vi>)
  n214 = control-ref of="参数下拉列表"() -> (w22:refnum<vi>)
  n215 = control-ref of="量程下拉列表"() -> (w23:refnum<vi>)
  n216 = control-ref of="备用系数"() -> (w18:refnum<vi>)
  n217 = control-ref of="公式"() -> (w20:refnum<vi>)
  n218 = while {
    tunnel: w41 -> [w392]
    tunnel: w42 -> [_]
    shift-right: [w386] -> _
    shift-left: enum16{"氨氮", "总磷"}."氨氮" ("枚举") -> [w387]
    stop <- FALSE stop-if-true
    w385 = u16 3 items=["总磷"=1, "氨氮"=3] ("站号")
    # "试剂填充 172 \n管路清洗108\n氨氮92\n总磷131\n总磷海水147\n总氮76\n总氮海水92"
    n219 = Wait (ms)(milliseconds to wait=u32 1000 ("等待时间（毫秒）")) -> ()  [unwired: 1 out]
    n220 = Bundle By Name(cluster=cluster{"命令":string, "data":variant} {"命令"="", "data"=variant} ("元素"), "命令"="读状态告警区", "data"=w385) -> (w394:cluster{"命令":string, "data":variant})
    n221 = global read "VAR总磷氨氮全局变量.vi" "状态告警区"() -> (w383:T4)
    n222 = Bundle By Name(cluster=cluster{"命令":string, "data":variant} {"命令"="", "data"=variant} ("元素"), "命令"="读测量数据区", "data"=w385) -> (w390:cluster{"命令":string, "data":variant})
    n223 = Unbundle By Name(w383) -> ("系统时间"=w382:timestamp)
    n224 = Enqueue Element(queue=w392, element=w394) -> (queue out=w388:refnum<queue>)  [unwired: 2 in, 2 out]
    n225 = Enqueue Element(queue=w388, element=w390) -> (queue out=w384:refnum<queue>)  [unwired: 2 in, 2 out]
    n226 = Get Date/Time In Seconds() -> (seconds since 1Jan1904=w381:timestamp)
    n227 = Subtract(x=w381, y=w382) -> (x-y=w380:dbl)
    n228 = Absolute Value(x=w380) -> (abs(x)=w379:dbl)
    n229 = global read "VAR总磷氨氮全局变量.vi" "通讯状态"() -> (w375:bool)
    n230 = Greater Or Equal?(x=w379, y=120.0) -> (x >= y?=w377:bool)
    n231 = And(x=w375, y=w377) -> (x .and. y?=w376:bool)
    n232 = case shown="真" w376 {
      tunnel: w384 -> [_ w399]
      frame False {
      }
      frame True {
        n233 = call "总磷氨氮启动命令.vi"("参数"=T5 {"站号"=3, "量程切换"=enum."AUTO", "控制命令"=enum."校时", "模式设置"=enum."待机", "测量间隔"=0}) -> ("启动命令"=w398:cluster{"命令":string, "data":variant})  [unwired: 10 in]
        n234 = Enqueue Element(queue=w399, element=w398) -> ()  [unwired: 2 in, 3 out]
      }
    }
    n235 = Increment(x=w387) -> (x+1=w386:enum16{"氨氮", "总磷"})
  }
  n236 = while {
    tunnel: w41 -> [w408]
    tunnel: w23 -> [w407]
    tunnel: w22 -> [w406]
    tunnel: w21 -> [w405]
    tunnel: w20 -> [w404]
    tunnel: w19 -> [w403]
    tunnel: w18 -> [w402]
    tunnel: w11 -> [w401]
    tunnel: w1 -> [_]
    stop <- FALSE stop-if-true
    n237 = event shown="[1] \"质控参数设置\": 值改变" {
      selector: _ -> [_ _ _ _ _ _ _ _ _ _ _ _ _ _ _ _ _ _ _]
      dyn-events: _ -> [_ _ _ _ _ _ _ _ _ _ _ _ _ _ _ _ _ _ _]
      timeout: _ -> [_ _ _ _ _ _ _ _ _ _ _ _ _ _ _ _ _ _ _]
      tunnel: w408 -> [_ _ _ w453 _ w478 w483 _ _ _ _ _ _ _ _ _ _ _ _]
      tunnel: w407 -> [_ _ _ _ _ _ _ _ _ _ _ _ _ w565 _ w585 w594 _ _]
      tunnel: w406 -> [_ _ _ _ _ _ _ _ _ _ _ _ _ w563 _ w583 w596 w604 w611]
      tunnel: w405 -> [_ _ _ _ _ _ _ _ _ _ _ _ _ w564 _ w584 w595 _ _]
      tunnel: w404 -> [_ _ _ _ _ _ _ _ _ _ _ _ _ w559 _ _ _ _ _]
      tunnel: w403 -> [_ _ _ _ _ _ _ _ _ _ _ _ _ _ _ w579 _ _ _]
      tunnel: w402 -> [_ _ _ _ _ _ _ _ _ _ _ _ _ _ _ _ _ w602 _]
      tunnel: w401 -> [_ _ _ _ _ _ w481 _ _ _ _ _ _ _ _ _ _ _ _]
      event Timeout {
        n238 = event-data() -> ()  [unwired: 1 in, 3 out]
      }
      event "质控参数设置": Value Change {
        n239 = event-data() -> ()  [unwired: 1 in, 6 out]
        n240 = global read "氨氮断电保存全局变量.vi" "质控参数设置"() -> (w410:T20)
        n241 = call "质控参数设置.vi"("质控参数设置"=w410) -> ("输出簇"=w411:T21)  [unwired: 10 in]
        n242 = Unbundle By Name(w411) -> ("确定"=w412:bool)
        n243 = case shown="真" w412 {
          tunnel: w411 -> [_ w414]
          tunnel: w410 -> [_ w413]
          frame False {
          }
          frame True {
            n244 = flat-sequence {
              tunnel: w414 -> [w421]
              tunnel: w413 -> [w415]
              frame #0 {
                n245 = Unbundle By Name(w421) -> ("跨度值"=w420:dbl, "零点标准液浓度"=w419:dbl, "跨度标准液浓度"=w418:dbl, "标准液标准浓度"=w417:dbl)
                n246 = Bundle By Name(cluster=w415, "跨度值"=w420, "零点标准液浓度"=w419, "跨度标准液浓度"=w418, "标准液标准浓度"=w417) -> (w416:T20)
                n247 = global write "氨氮断电保存全局变量.vi" "质控参数设置"(w416) -> ()
              }
              frame #1 {
                n248 = call <vilib>:"Application Directory.vi"() -> ("Application Directory"=w422:path)
                n249 = Build Path(base path=w422, name or relative path="data\\sys.ini" ("名称或相对路径")) -> (appended path=w424:path)
                n250 = call <vilib>:"Open Config Data.vi"("configuration file path"=w424) -> ("error out"=w428:errorcluster, "refnum"=w425:T18)  [unwired: 8 in, 1 out]
                n251 = vi-ref "氨氮.lvlib:氨氮断电保存全局变量.vi"() -> (w426:refnum<vi>)
                n252 = call <userlib>:"Write Panel to INI__ogtk.vi"("error in (no error)"=w428, "VI ref"=w426, "refnum"=w425) -> ("error out"=w429:errorcluster, "refnum out"=w427:T18)  [unwired: 7 in]
                n253 = call <vilib>:"Close Config Data.vi"("error in (no error)"=w429, "refnum"=w427) -> ("error out"=w434:errorcluster, "file path"=w435:path)  [unwired: 8 in]
                n254 = Open/Create/Replace File(file path (use dialog)=w435, error in=w434) -> (refnum out=w431:refnum<file>, error out=w430:errorcluster)  [unwired: 4 in, 1 out]
                n255 = Flush File(refnum=w431, error in=w430) -> (refnum out=w432:refnum<file>, error out=w433:errorcluster)
                n256 = Close File(refnum=w432, error in=w433) -> ()  [unwired: 2 out]
              }
            }
          }
        }
      }
      event "氨氮自动测试量程配置": Value Change {
        n257 = event-data() -> ()  [unwired: 1 in, 6 out]
        n258 = flat-sequence {
          frame #0 {
            n259 = global write "氨氮断电保存全局变量.vi" "氨氮自动测试量程配置"("氨氮自动测试量程配置") -> ()
          }
          frame #1 {
            n260 = call <vilib>:"Application Directory.vi"() -> ("Application Directory"=w450:path)
            n261 = Build Path(base path=w450, name or relative path="data\\sys.ini" ("名称或相对路径")) -> (appended path=w448:path)
            n262 = call <vilib>:"Open Config Data.vi"("configuration file path"=w448) -> ("error out"=w444:errorcluster, "refnum"=w447:T18)  [unwired: 8 in, 1 out]
            n263 = vi-ref "氨氮.lvlib:氨氮断电保存全局变量.vi"() -> (w446:refnum<vi>)
            n264 = call <userlib>:"Write Panel to INI__ogtk.vi"("error in (no error)"=w444, "VI ref"=w446, "refnum"=w447) -> ("error out"=w443:errorcluster, "refnum out"=w445:T18)  [unwired: 7 in]
            n265 = call <vilib>:"Close Config Data.vi"("error in (no error)"=w443, "refnum"=w445) -> ("error out"=w438:errorcluster, "file path"=w437:path)  [unwired: 8 in]
            n266 = Open/Create/Replace File(file path (use dialog)=w437, error in=w438) -> (refnum out=w441:refnum<file>, error out=w442:errorcluster)  [unwired: 4 in, 1 out]
            n267 = Flush File(refnum=w441, error in=w442) -> (refnum out=w440:refnum<file>, error out=w439:errorcluster)
            n268 = Close File(refnum=w440, error in=w439) -> ()  [unwired: 2 out]
          }
        }
      }
      event "手动启动": Value Change {
        n269 = event-data() -> ()  [unwired: 1 in, 6 out]
        n270 = call "总磷氨氮启动参数对话框.vi"() -> ("确认"=w451:bool, "元素"=w452:cluster{"命令":string, "data":variant})  [unwired: 10 in]
        n271 = case shown="真" w451 {
          tunnel: w453 -> [_ w455]
          tunnel: w452 -> [_ w454]
          frame False {
          }
          frame True {
            n272 = Enqueue Element(queue=w455, element=w454) -> ()  [unwired: 2 in, 3 out]
          }
        }
      }
      event "定时启动": Mouse Down {
        n273 = event-data() -> ()  [unwired: 1 in, 6 out]
        n274 = flat-sequence {
          frame #0 {
            n275 = global read "氨氮断电保存全局变量.vi" "定时控制"() -> (w456:T7)
            n276 = call "周期设置.vi"("定时控制参数输入"=w456) -> ("定时控制参数输出"=w457:T7)  [unwired: 10 in]
            n277 = global write "氨氮断电保存全局变量.vi" "定时控制"(w457) -> ()
          }
          frame #1 {
            n278 = call <vilib>:"Application Directory.vi"() -> ("Application Directory"=w471:path)
            n279 = Build Path(base path=w471, name or relative path="data\\sys.ini" ("名称或相对路径")) -> (appended path=w469:path)
            n280 = call <vilib>:"Open Config Data.vi"("configuration file path"=w469) -> ("error out"=w465:errorcluster, "refnum"=w468:T18)  [unwired: 8 in, 1 out]
            n281 = vi-ref "氨氮.lvlib:氨氮断电保存全局变量.vi"() -> (w467:refnum<vi>)
            n282 = call <userlib>:"Write Panel to INI__ogtk.vi"("error in (no error)"=w465, "VI ref"=w467, "refnum"=w468) -> ("error out"=w464:errorcluster, "refnum out"=w466:T18)  [unwired: 7 in]
            n283 = call <vilib>:"Close Config Data.vi"("error in (no error)"=w464, "refnum"=w466) -> ("error out"=w459:errorcluster, "file path"=w458:path)  [unwired: 8 in]
            n284 = Open/Create/Replace File(file path (use dialog)=w458, error in=w459) -> (refnum out=w462:refnum<file>, error out=w463:errorcluster)  [unwired: 4 in, 1 out]
            n285 = Flush File(refnum=w462, error in=w463) -> (refnum out=w461:refnum<file>, error out=w460:errorcluster)
            n286 = Close File(refnum=w461, error in=w460) -> ()  [unwired: 2 out]
          }
        }
      }
      event "单步测试": Value Change {
        w473 = u16 1 items=["总磷"=1, "氨氮"=3] ("站号")
        n287 = event-data() -> ()  [unwired: 1 in, 6 out]
        n288 = Bundle("站号"=w473, "总磷氨氮调试"="总磷氨氮调试") -> (w472:cluster{"站号":u16, "总磷氨氮调试":u16[]})  [unwired: 1 in]
        n289 = Bundle By Name(cluster=cluster{"命令":string, "data":variant} {"命令"="", "data"=variant} ("元素"), "命令"="debug", "data"=w472) -> (w475:cluster{"命令":string, "data":variant})
        n290 = Enqueue Element(queue=w478, element=w475) -> ()  [unwired: 2 in, 3 out]
      }
      event "停止": Value Change {
        n291 = event-data() -> ()  [unwired: 1 in, 6 out]
        n292 = Enqueue Element(queue=w483, element=cluster{"命令":string, "data":variant} {"命令"="启动", "data"=variant(cluster{"站号":u16, "控制命令输出":u16[]} {"站号"=3, "控制命令输出"=[2816]})} ("启动命令")) -> ()  [unwired: 2 in, 3 out]
        n293 = Cancel Notification(0:w481) -> (8:w480:refnum<notifier>)  [unwired: 1 in, 2 out]
        n294 = Send Notification(notification=TRUE ("通知"), notifier=w480) -> ()  [unwired: 1 in, 2 out]
      }
      event "设置": Value Change {
        n295 = event-data() -> ()  [unwired: 1 in, 6 out]
        n296 = property on="窗格" class="Pane"("Origin"=T10 {"Horizontal"=0, "Vertical"=628} ("原点")) -> ()  [unwired: 2 in, 2 out]
      }
      event "返回": Value Change {
        n297 = event-data() -> ()  [unwired: 1 in, 6 out]
        n298 = property on="窗格" class="Pane"("Origin"=T10 {"Horizontal"=0, "Vertical"=0} ("原点")) -> ()  [unwired: 2 in, 2 out]
      }
      event "标液浓度1", "测量吸光度1", "测量吸光度2", "标液浓度2", "测量吸光度3", "标液浓度3", "测量吸光度4", "标液浓度4", "测量吸光度5", "标液浓度5", "样品1启用", "样品3启用", "样品4启用", "样品5启用", "样品2启用", "模型", "method", "精度": Value Change {
        n299 = event-data() -> ()  [unwired: 1 in, 6 out]
        n300 = flat-sequence {
          frame #0 {
            n301 = Replace Array Subset(array=dbl[] [0.0, 0.0, 0.0, 0.0, 0.0] ("数组"), new element #1="标液浓度1", new element #2="标液浓度2", new element #3="标液浓度3", new element #4="标液浓度4", new element #5="标液浓度5") -> (w511:dbl[])  [unwired: 5 in]
            n302 = Replace Array Subset(array=dbl[] [0.0, 0.0, 0.0, 0.0, 0.0] ("数组"), new element #1="测量吸光度1", new element #2="测量吸光度2", new element #3="测量吸光度3", new element #4="测量吸光度4", new element #5="测量吸光度5") -> (w510:dbl[])  [unwired: 5 in]
            n303 = Replace Array Subset(array=bool[] [FALSE, FALSE, FALSE, FALSE, FALSE] ("数组"), new element #1="样品1启用", new element #2="样品2启用", new element #3="样品3启用", new element #4="样品4启用", new element #5="样品5启用") -> (w509:bool[])  [unwired: 5 in]
            n304 = call "线性公式.vi"("精度"="精度", "模型"="模型", "method"="method", "启用"=w509, "监测浓度"=w510, "标液浓度"=w511) -> ("XY图"=w506:cluster{"X Values":dbl[], "Y Values":dbl[]}[], "r^2"=w489:dbl, "拟合方程"=w490:string)  [unwired: 3 in]
            "XY图" <- w506
            "拟合公式" <- w490
            "r^2" <- w489
            n305 = global read "氨氮断电保存全局变量.vi" "曲线模型"() -> (w508:T19)
            n306 = Bundle By Name(cluster=w508, "XY图"=w506, "标液浓度1"="标液浓度1", "测量吸光度1"="测量吸光度1", "测量吸光度2"="测量吸光度2", "标液浓度2"="标液浓度2", "测量吸光度3"="测量吸光度3", "标液浓度3"="标液浓度3", "测量吸光度4"="测量吸光度4", "标液浓度4"="标液浓度4", "测量吸光度5"="测量吸光度5", "标液浓度5"="标液浓度5", "样品1启用"="样品1启用", "样品3启用"="样品3启用", "样品4启用"="样品4启用", "样品5启用"="样品5启用", "样品2启用"="样品2启用", "拟合公式"=w490, "r^2"=w489, "模型"="模型", "method"="method", "精度"="精度") -> (w507:T19)
            n307 = global write "氨氮断电保存全局变量.vi" "曲线模型"(w507) -> ()
          }
          frame #1 {
            n308 = call <vilib>:"Application Directory.vi"() -> ("Application Directory"=w528:path)
            n309 = Build Path(base path=w528, name or relative path="data\\sys.ini" ("名称或相对路径")) -> (appended path=w526:path)
            n310 = call <vilib>:"Open Config Data.vi"("configuration file path"=w526) -> ("error out"=w523:errorcluster, "refnum"=w525:T18)  [unwired: 8 in, 1 out]
            n311 = vi-ref "氨氮.lvlib:氨氮断电保存全局变量.vi"() -> (w515:refnum<vi>)
            n312 = call <userlib>:"Write Panel to INI__ogtk.vi"("error in (no error)"=w523, "VI ref"=w515, "refnum"=w525) -> ("error out"=w522:errorcluster, "refnum out"=w524:T18)  [unwired: 7 in]
            n313 = call <vilib>:"Close Config Data.vi"("error in (no error)"=w522, "refnum"=w524) -> ("error out"=w517:errorcluster, "file path"=w516:path)  [unwired: 8 in]
            n314 = Open/Create/Replace File(file path (use dialog)=w516, error in=w517) -> (refnum out=w520:refnum<file>, error out=w521:errorcluster)  [unwired: 4 in, 1 out]
            n315 = Flush File(refnum=w520, error in=w521) -> (refnum out=w519:refnum<file>, error out=w518:errorcluster)
            n316 = Close File(refnum=w519, error in=w518) -> ()  [unwired: 2 out]
          }
        }
      }
      event "样品1 F0", "样品1 F1", "样品2 F1", "样品2 F0", "样品3 F1", "样品3 F0", "样品4 F0", "样品4 F1", "样品5 F1", "样品5 F0": Value Change {
        n317 = event-data() -> ()  [unwired: 1 in, 6 out]
        n318 = global read "氨氮断电保存全局变量.vi" "曲线模型"() -> (w540:T19)
        n319 = formula code="E=log(F0/F1);"("F0"="样品1 F0", "F1"="样品1 F1") -> ("E"=w545:dbl)
        n320 = formula code="E=log(F0/F1);"("F0"="样品2 F0", "F1"="样品2 F1") -> ("E"=w544:dbl)
        n321 = formula code="E=log(F0/F1);"("F0"="样品3 F0", "F1"="样品3 F1") -> ("E"=w543:dbl)
        n322 = formula code="E=log(F0/F1);"("F0"="样品4 F0", "F1"="样品4 F1") -> ("E"=w542:dbl)
        n323 = formula code="E=log(F0/F1);"("F0"="样品5 F0", "F1"="样品5 F1") -> ("E"=w541:dbl)
        n324 = Bundle By Name(cluster=w540, "样品1 F0"="样品1 F0", "样品1 F1"="样品1 F1", "样品2 F1"="样品2 F1", "样品2 F0"="样品2 F0", "样品3 F1"="样品3 F1", "样品3 F0"="样品3 F0", "样品4 F0"="样品4 F0", "样品4 F1"="样品4 F1", "样品5 F1"="样品5 F1", "样品5 F0"="样品5 F0") -> (w539:T19)
        n325 = global write "氨氮断电保存全局变量.vi" "曲线模型"(w539) -> ()
        n326 = property on="测量吸光度1" class="DigNum (严格)"("Val(Sgnl)"=w545) -> ()  [unwired: 2 in, 2 out]
        n327 = property on="测量吸光度2" class="DigNum (严格)"("Val(Sgnl)"=w544) -> ()  [unwired: 2 in, 2 out]
        n328 = property on="测量吸光度3" class="DigNum (严格)"("Val(Sgnl)"=w543) -> ()  [unwired: 2 in, 2 out]
        n329 = property on="测量吸光度4" class="DigNum (严格)"("Val(Sgnl)"=w542) -> ()  [unwired: 2 in, 2 out]
        n330 = property on="测量吸光度5" class="DigNum (严格)"("Val(Sgnl)"=w541) -> ()  [unwired: 2 in, 2 out]
      }
      event "标液浓度1", "标液浓度2", "标液浓度3", "标液浓度4", "标液浓度5", "样品1 F0", "样品1 F1", "样品2 F1", "样品2 F0", "样品3 F1", "样品3 F0", "样品4 F0", "样品4 F1", "样品5 F0", "样品5 F1", "精度", "公式.X^2", "公式.X", "公式.b", "量程切换阈值.阈值", "量程切换阈值.标液浓度", "备用系数.量程上限", "备用系数.量程下限", "备用系数.检出限", "备用系数.精度": Mouse Down {
        n331 = event-data() -> ("CtlRef"=w549:refnum<vi>)  [unwired: 1 in, 5 out]
        n332 = property class="DigNum (严格)"(reference=w549) -> (reference out=w547:refnum<vi>, "Value"=w548:dbl)  [unwired: 1 in, 1 out]
        n333 = call "数字键盘.vi"("OldNumber"=w548) -> ("NewNumber"=w546:dbl)
        n334 = property class="DigNum (严格)"(reference=w547, "Val(Sgnl)"=w546) -> ()  [unwired: 1 in, 2 out]
      }
      event "测量吸光度1", "测量吸光度2", "测量吸光度3", "测量吸光度4", "测量吸光度5": Mouse Down {
        n335 = event-data() -> ("CtlRef"=w553:refnum<vi>)  [unwired: 1 in, 7 out]
        n336 = property class="DigNum (严格)"(reference=w553) -> (reference out=w554:refnum<vi>, "Value"=w551:dbl)  [unwired: 1 in, 1 out]
        n337 = call "数字键盘.vi"("OldNumber"=w551) -> ("NewNumber"=w552:dbl)
        n338 = property class="DigNum (严格)"(reference=w554, "Val(Sgnl)"=w552) -> ()  [unwired: 1 in, 2 out]
        n339 = Not Equal?(x=w552, y=w551) -> (x != y?=w550:bool)
        n340 = case shown="真" w550 {
          frame False {
          }
          frame True {
            w555 = 0.0 ("样品1 F0")
            n341 = local write "样品1 F1"(w555) -> ()
            n342 = local write "样品2 F0"(w555) -> ()
            n343 = local write "样品2 F1"(w555) -> ()
            n344 = local write "样品3 F0"(w555) -> ()
            n345 = local write "样品3 F1"(w555) -> ()
            n346 = local write "样品4 F0"(w555) -> ()
            n347 = local write "样品4 F1"(w555) -> ()
            n348 = local write "样品5 F0"(w555) -> ()
            n349 = local write "样品5 F1"(w555) -> ()
            n350 = local write "样品1 F0"(w555) -> ()
          }
        }
      }
      event "读公式": Value Change {
        n351 = event-data() -> ()  [unwired: 1 in, 6 out]
        n352 = property class="Enum (严格)"(reference=w563) -> ("Value"=w562:enum16{"氨氮", "总磷"})  [unwired: 1 in, 2 out]
        n353 = property class="Enum (严格)"(reference=w564) -> ("Value"=w561:enum16{"水样测量", "空白核查", "跨度核查", "标样核查", "加标回收"})  [unwired: 1 in, 2 out]
        n354 = property class="Enum (严格)"(reference=w565) -> ("Value"=w560:enum16{"低量程", "高量程"})  [unwired: 1 in, 2 out]
        n355 = call "总磷氨氮公式读取.vi"("量程"=w560, "测量模式"=w561, "测量参数"=w562) -> ("error out"=w557:errorcluster, "公式"=w558:cluster{"X^2":dbl, "X":dbl, "b":dbl})  [unwired: 7 in]
        n356 = property class="Clust (严格)"(reference=w559, "Value"=w558) -> ()  [unwired: 1 in, 2 out]
        n357 = case shown="错误" w557 {
          tunnel: ["读取成功" ("消息") "读取失败" ("消息")] -> w556
          frame No Error {
          }
          frame Error {
          }
        }
        n358 = One Button Dialog(message=w556) -> ()  [unwired: 1 in, 1 out]
      }
      event "写公式": Value Change {
        n359 = event-data() -> ()  [unwired: 1 in, 6 out]
        n360 = call "总磷氨氮公式写入.vi"("公式"="公式", "量程"="量程下拉列表", "测量模式"="测量模式下拉列表", "测量参数"="参数下拉列表") -> ("error out"=w568:errorcluster)  [unwired: 7 in]
        n361 = case shown="无错误" w568 {
          tunnel: ["写入成功" ("消息") "写入失败" ("消息")] -> w569
          frame No Error {
          }
          frame Error {
          }
        }
        n362 = One Button Dialog(message=w569) -> ()  [unwired: 1 in, 1 out]
      }
      event "量程切换阈值读取": Value Change {
        n363 = event-data() -> ()  [unwired: 1 in, 6 out]
        n364 = property class="Enum (严格)"(reference=w583) -> ("Value"=w582:enum16{"氨氮", "总磷"})  [unwired: 1 in, 2 out]
        n365 = property class="Enum (严格)"(reference=w584) -> ("Value"=w581:enum16{"水样测量", "空白核查", "跨度核查", "标样核查", "加标回收"})  [unwired: 1 in, 2 out]
        n366 = property class="Enum (严格)"(reference=w585) -> ("Value"=w580:enum16{"低量程", "高量程"})  [unwired: 1 in, 2 out]
        n367 = call "总磷氨氮量程读取.vi"("量程"=w580, "测量模式"=w581, "测量参数"=w582) -> ("error out"=w576:errorcluster, "量程切换阈值"=w578:cluster{"阈值":dbl, "标液浓度":dbl})  [unwired: 7 in]
        n368 = property class="Clust (严格)"(reference=w579, "Value"=w578) -> ()  [unwired: 1 in, 2 out]
        n369 = case shown="错误" w576 {
          tunnel: ["读取成功" ("消息") "读取失败" ("消息")] -> w577
          frame No Error {
          }
          frame Error {
          }
        }
        n370 = One Button Dialog(message=w577) -> ()  [unwired: 1 in, 1 out]
      }
      event "量程切换阈值写入": Value Change {
        n371 = event-data() -> ()  [unwired: 1 in, 6 out]
        n372 = property class="Enum (严格)"(reference=w596) -> ("Value"=w593:enum16{"氨氮", "总磷"})  [unwired: 1 in, 2 out]
        n373 = property class="Enum (严格)"(reference=w595) -> ("Value"=w592:enum16{"水样测量", "空白核查", "跨度核查", "标样核查", "加标回收"})  [unwired: 1 in, 2 out]
        n374 = property class="Enum (严格)"(reference=w594) -> ("Value"=w591:enum16{"低量程", "高量程"})  [unwired: 1 in, 2 out]
        n375 = call "总磷氨氮量程写入.vi"("量程切换阈值"="量程切换阈值", "量程"=w591, "测量模式"=w592, "测量参数"=w593) -> ("error out"=w588:errorcluster)  [unwired: 7 in]
        n376 = case shown="无错误" w588 {
          tunnel: ["写入成功" ("消息") "写入失败" ("消息")] -> w589
          frame No Error {
          }
          frame Error {
          }
        }
        n377 = One Button Dialog(message=w589) -> ()  [unwired: 1 in, 1 out]
      }
      event "备用系数读取": Value Change {
        n378 = event-data() -> ()  [unwired: 1 in, 6 out]
        n379 = property class="Enum (严格)"(reference=w604) -> ("Value"=w603:enum16{"氨氮", "总磷"})  [unwired: 1 in, 2 out]
        n380 = call "总磷氨氮备用系数读取.vi"("测量参数"=w603) -> ("error out"=w599:errorcluster, "备用系数"=w601:T2)  [unwired: 9 in]
        n381 = property class="Clust (严格)"(reference=w602, "Value"=w601) -> ()  [unwired: 1 in, 2 out]
        n382 = case shown="错误" w599 {
          tunnel: ["读取成功" ("消息") "读取失败" ("消息")] -> w600
          frame No Error {
          }
          frame Error {
          }
        }
        n383 = One Button Dialog(message=w600) -> ()  [unwired: 1 in, 1 out]
      }
      event "备用系数写入": Value Change {
        n384 = event-data() -> ()  [unwired: 1 in, 6 out]
        n385 = property class="Enum (严格)"(reference=w611) -> ("Value"=w610:enum16{"氨氮", "总磷"})  [unwired: 1 in, 2 out]
        n386 = call "总磷氨氮备用系数写入.vi"("备用系数"="备用系数", "测量参数"=w610) -> ("error out"=w607:errorcluster)  [unwired: 9 in]
        n387 = case shown="无错误" w607 {
          tunnel: ["写入成功" ("消息") "写入失败" ("消息")] -> w608
          frame No Error {
          }
          frame Error {
          }
        }
        n388 = One Button Dialog(message=w608) -> ()  [unwired: 1 in, 1 out]
      }
    }
  }
